vi "EVO_main_raw_dev_MQTTT_RT_raw.vi"() -> ()   [LabVIEW 2017]
uses:
  controls/FPGA State.ctl
  mqtt Folder/src/class/mqtt/mqttTypedef/mqttConnectionStatus.ctl
  mqtt Folder/src/class/mqtt/mqttTypedef/mqttConnectionMeta.ctl
  mqtt Folder/src/class/mqtt/mqttTypedef/mqttQOSlevel.ctl
  controls/UI Data2.ctl
  mqtt Folder/src/class/mqtt/mqttTXqueue/mqttTXdataQueueFunction.ctl
  mqtt Folder/src/class/mqtt/mqttConfigFunction.ctl
  mqtt Folder/src/class/mqtt/mqttTypedef/mqttConnectionFlags.ctl
  mqtt Folder/src/class/mqtt/mqttTypedef/mqttWillInformation.ctl
  mqtt Folder/src/class/mqtt/mqttTypedef/mqttBroker.ctl
  controls/Chatter data.ctl
  <vilib>/addons/database/Connection.llb/DB Tools Open Connec (Path).vi
  Globals/Global - All UI Loop Stop.vi
  Globals/Global - UI Stream and Variable Connections.vi
  Globals/Global - Configuration Options.vi
  UI Error Handlers/support/User Event - Stop/User Event - Stop.lvlib
  UI Error Handlers/support/Message Queue/Message Queue.lvlib
  mqtt Folder/src/class/mqtt/mqtt.lvclass
  <vilib>/addons/database/NI_Database_API.lvlib
panel:
  out "size(s) 2":i32
  out "size(s)":i32
  out "publishSuccess":bool=TRUE
  out "publishMessageID":u16 format="%02x"
  in  "connMeta":T1
  in  "topic":string="a/b"
  out "connStatus 2":T3
  out "success":bool
  out "sessionPresent 2":bool
  in  "error in (no error)":errorcluster
  out "tag spike":string
  out "string":string
  out "x .or. y?":bool
  out "resulting string":string
  in  "Settings Tab":T4(tab)=enum."Sensor data "
  in  "Database_machine":string="Raw.DMG_MORI_DMU_40_EVO_RAW"
  in  "OK Button":bool
  in  "Tool Data File":path=path "K:/Core Research/Project Folders/AI Projects/AI3190 Digital Shop Floor Rollout/5 Software Files/Catapult/tool_path.txt"
  in  "Run Control":bool
  in  "Stop Control":bool
  in  "Max Acceleration Threshold (g)":sgl=0.03
  in  "In-cut Power Threshold":dbl=1.0
  in  "Controller Address":string="127.22.11.2"
  in  "Connect to Controller":bool
  out "Connected?":bool
  out "System Status":string
  in  "Save?":bool
  in  "Switch to Safe State":bool
  out "Current FPGA State":T5
  out "Tool Data":string="\n"
  in  "ODBC data source name":string="amrc_monitoring"
  in  "MT Connect Agent":string="http://amrcmtconnect.shef.ac.uk:5000/"
  in  "milliseconds to wait":u32=100
  in  "Machine":string="DMU40EVO"
  out "Loop execution":u32
  out "output cluster":cluster{"G1 ":bool}
  out "Chatter?":bool
  out "Automated FRF  (grms) 2":T6(graph)
  out "ACC  (grms)":T7(graph)
  out "Strain (grms)":T8(graph)
  out "Raw ACC":waveform(dbl)[](graph)
  out "Raw Waveform 2":waveform(dbl)[](graph)
  out "tag acc":string
  out "Feed rate":dbl[](graph)
  out "Spindle Speed":dbl[](graph)
  out "Spindle Load":dbl[](graph)
  out "H5 machine":bool
  out "Tool id":string
  out "RPM":dbl
  out "Program Name":string
  out "Block of code being executed":string
  out "Feed":dbl
  out "CPU Usage (%)":dbl[][](graph)
  out "Free Physical Memory or Largest Contiguous Memory (bytes)":dbl(graph)
  out "DMA FIFO Overflow?":bool
  in  "Exit":bool
  # "Acceleration Waveform for 0.5s"
  # "Connection Settings"
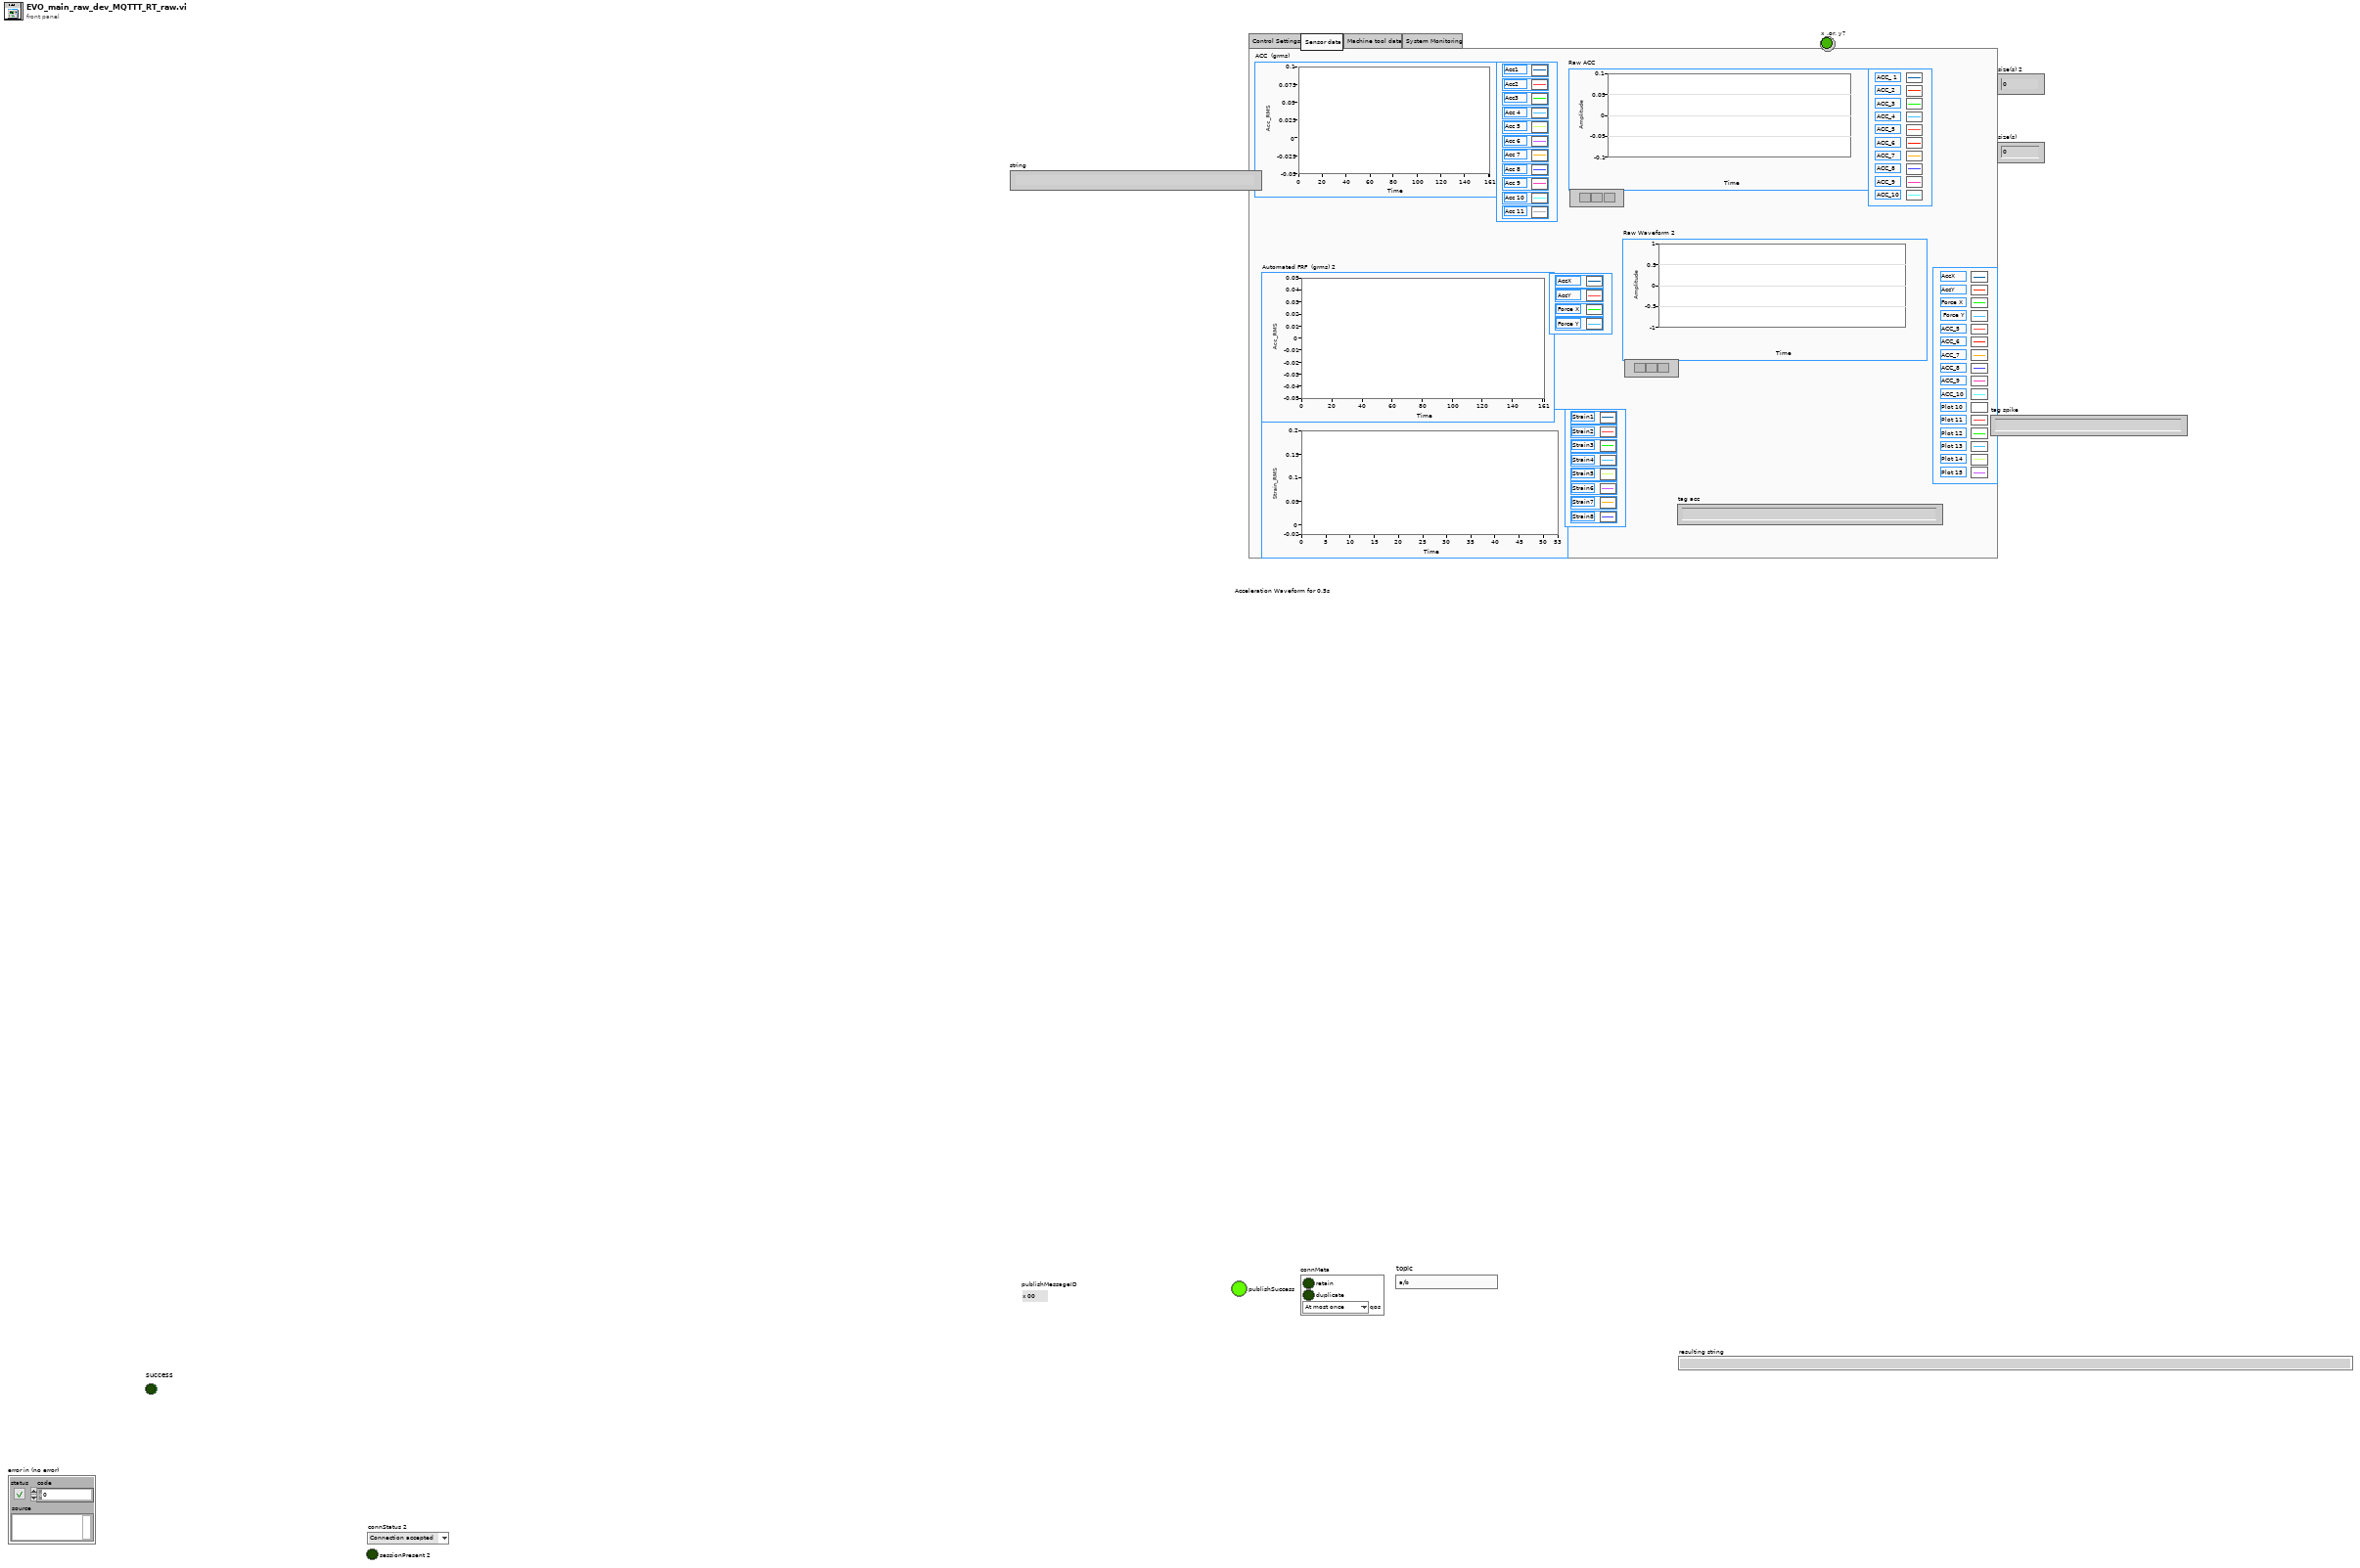
[diagram p1: front panel]
types:
  T1 = typedef "mqttConnectionMeta.ctl" = cluster{"retain":bool, "duplicate":bool, "qos":T2}
  T2 = typedef "mqttQOSlevel.ctl" = enum8{"At most once", "At least once", "Exactly once", "Reserved"}
  T3 = typedef "mqttConnectionStatus.ctl" = enum16{"Connection accepted", "Connection refused: unacceptable protocol version", "Connection refused: identifier rejected", "Connection refused: Server unavailable", "Connection refused: bad user name or password", "Connection refused: not authorized"}
  T4 = enum32{"Control Settings", "Sensor data ", "Machine tool data", "System Monitoring"}
  T5 = typedef "FPGA State.ctl" = enum16{"Safe State", "Control (PID)"}
  T6 = cluster{"[0]":dbl, "[1]":dbl, "[2]":dbl, "[3]":dbl}
  T7 = cluster{"[0]":dbl, "[1]":dbl, "[2]":dbl, "[3]":dbl, "[4]":dbl, "[5]":dbl, "[6]":dbl, "[7]":dbl, "[8]":dbl, "[9]":dbl, "[10]":dbl}
  T8 = cluster{"[0]":dbl, "[1]":dbl, "[2]":dbl, "[3]":dbl, "[4]":dbl, "[5]":dbl}
  T9 = typedef "mqttBroker.ctl" = cluster{"address":string, "port":u16, "connTimeout":i32, "writeTimeout":i32, "readTimeout":i32, "subTimeout":i32}
  T10 = typedef "mqttWillInformation.ctl" = cluster{"User Name":string, "Password":string}
  T11 = typedef "mqttConnectionFlags.ctl" = cluster{"reserved":bool, "clean session":bool, "will flag":bool, "willQOS":enum8{"At most once", "At least once", "Exactly once", "Reserved"}, "will retain":bool, "password":bool, "user name":bool}
  T12 = typedef "mqtt.lvclass/mqttConfigFunction.ctl" = enum16{"init", "deinit", "set", "get"}
  T13 = enum8{"Enabled", "Disabled", "Disabled and Grayed Out"}
  T14 = typedef "mqttTXdataQueueFunction.ctl" = enum16{"init", "deinit", "getQueue", "enqueue"}
  T15 = typedef "UI Data2.ctl" = cluster{"Switch to Safe State Ref":refnum<vi>, "Run Control Ref":refnum<vi>, "Stop Control Ref":refnum<vi>, "Update Control Configurations Ref":refnum<vi>, "Chatter Data Ref":refnum<vi>, "Max Acceleration Threshold Ref":refnum<vi>}
  T16 = typedef "NI_Database_API.lvlib/Conn ObjectReference.ctl" = refnum<k1>
  T17 = typedef "Message Queue.lvlib/All Message Queues.ctl" = cluster{"UI":refnum<queue>}
  T18 = cluster{"Message":string, "Message Data":variant}
  T19 = typedef "Chatter data.ctl" = cluster{"Tool data":cluster{"Number of teeth":sgl}, "Cutting data":cluster{"rpm":sgl}, "Limits":cluster{"Magnitude threshold":sgl, "Tolerance":sgl}, "G1 status":cluster{"G1 ":bool}}
  T20 = cluster{"FPGA State":T5, "Max Acceleration Threshold":sgl, "Chatter Data":T19}
  T21 = cluster{"seconds since 1Jan1904":timestamp, "number":dbl[][], "Machine Data":cluster{"Zload":string, "Yload":string, "Xload":string, "path_position":string, "Fovr":string, "SspeedOvr":string, "Program Name":string, "Program status":string, "Block of code being executed":string, "Line of code":string, "Machine availability":string, "Emergency status":string, "Controller mode":string, "Tool_id":string}}
  T22 = cluster{"seconds since 1Jan1904":timestamp, "number":dbl[][], "Machine Data":cluster{"Zload":string, "Yload":string, "Xload":string, "path_position":string, "Fovr":string, "SspeedOvr":string, "Program Name":string, "Program status":string, "Block of code being executed":string, "Line of code":string, "Machine availability":string, "Emergency status":string, "Controller mode":string, "Tool id":string}}
  T23 = cluster{"Actual PID Loop Period":refnum<k21>, "DMA FIFO Overflow?":refnum<k21>, "CPU Usage":refnum<k21>, "Free or Contiguous Memory":refnum<k21>, "Current FPGA State":refnum<k21>, "Acceleration (grms)":refnum<k21>, "Acceleration Waveform":refnum<k21>, "Chatter":refnum<k21>, "tag acc":refnum<k21>, "tag video":refnum<k21>, "Image Waveform":refnum<k21>}
  T24 = cluster{"Zload":string, "Yload":string, "Xload":string, "path_position":string, "Fovr":string, "SspeedOvr":string, "Program Name":string, "Program status":string, "Block of code being executed":string, "Line of code":string, "Machine availability":string, "Emergency status":string, "Controller mode":string, "Tool_id":string}
  T25 = cluster{"Zload":string, "Yload":string, "Xload":string, "path_position":string, "Fovr":string, "SspeedOvr":string, "Program Name":string, "Program status":string, "Block of code being executed":string, "Line of code":string, "Machine availability":string, "Emergency status":string, "Controller mode":string, "Tool id":string}
  T26 = cluster{"Magnitude threshold":sgl, "Tolerance":sgl}
  T27 = typedef "FPGA state.ctl" = enum16{"Safe State", "Control (PID)"}
  T28 = typedef "IMAQ Image.ctl" = refnum<image>
  T29 = typedef "CPU Loads.ctl" = cluster{"Total (%)":dbl, "Time Critical (%)":dbl, "Timed Structures (%)":dbl, "High (%)":dbl, "Above Normal (%)":dbl, "Normal (%)":dbl, "Background (%)":dbl, "Idle (%)":dbl, "ISR (%)":dbl}[]
  T30 = cluster{"seconds since 1Jan1904":timestamp, "appended array":dbl[][], "Machine Data":cluster{"Zload":string, "Yload":string, "Xload":string, "path_position":string, "Fovr":string, "SspeedOvr":string, "Program Name":string, "Program status":string, "Block of code being executed":string, "Line of code":string, "Machine availability":string, "Emergency status":string, "Controller mode":string, "Tool_id":string}}
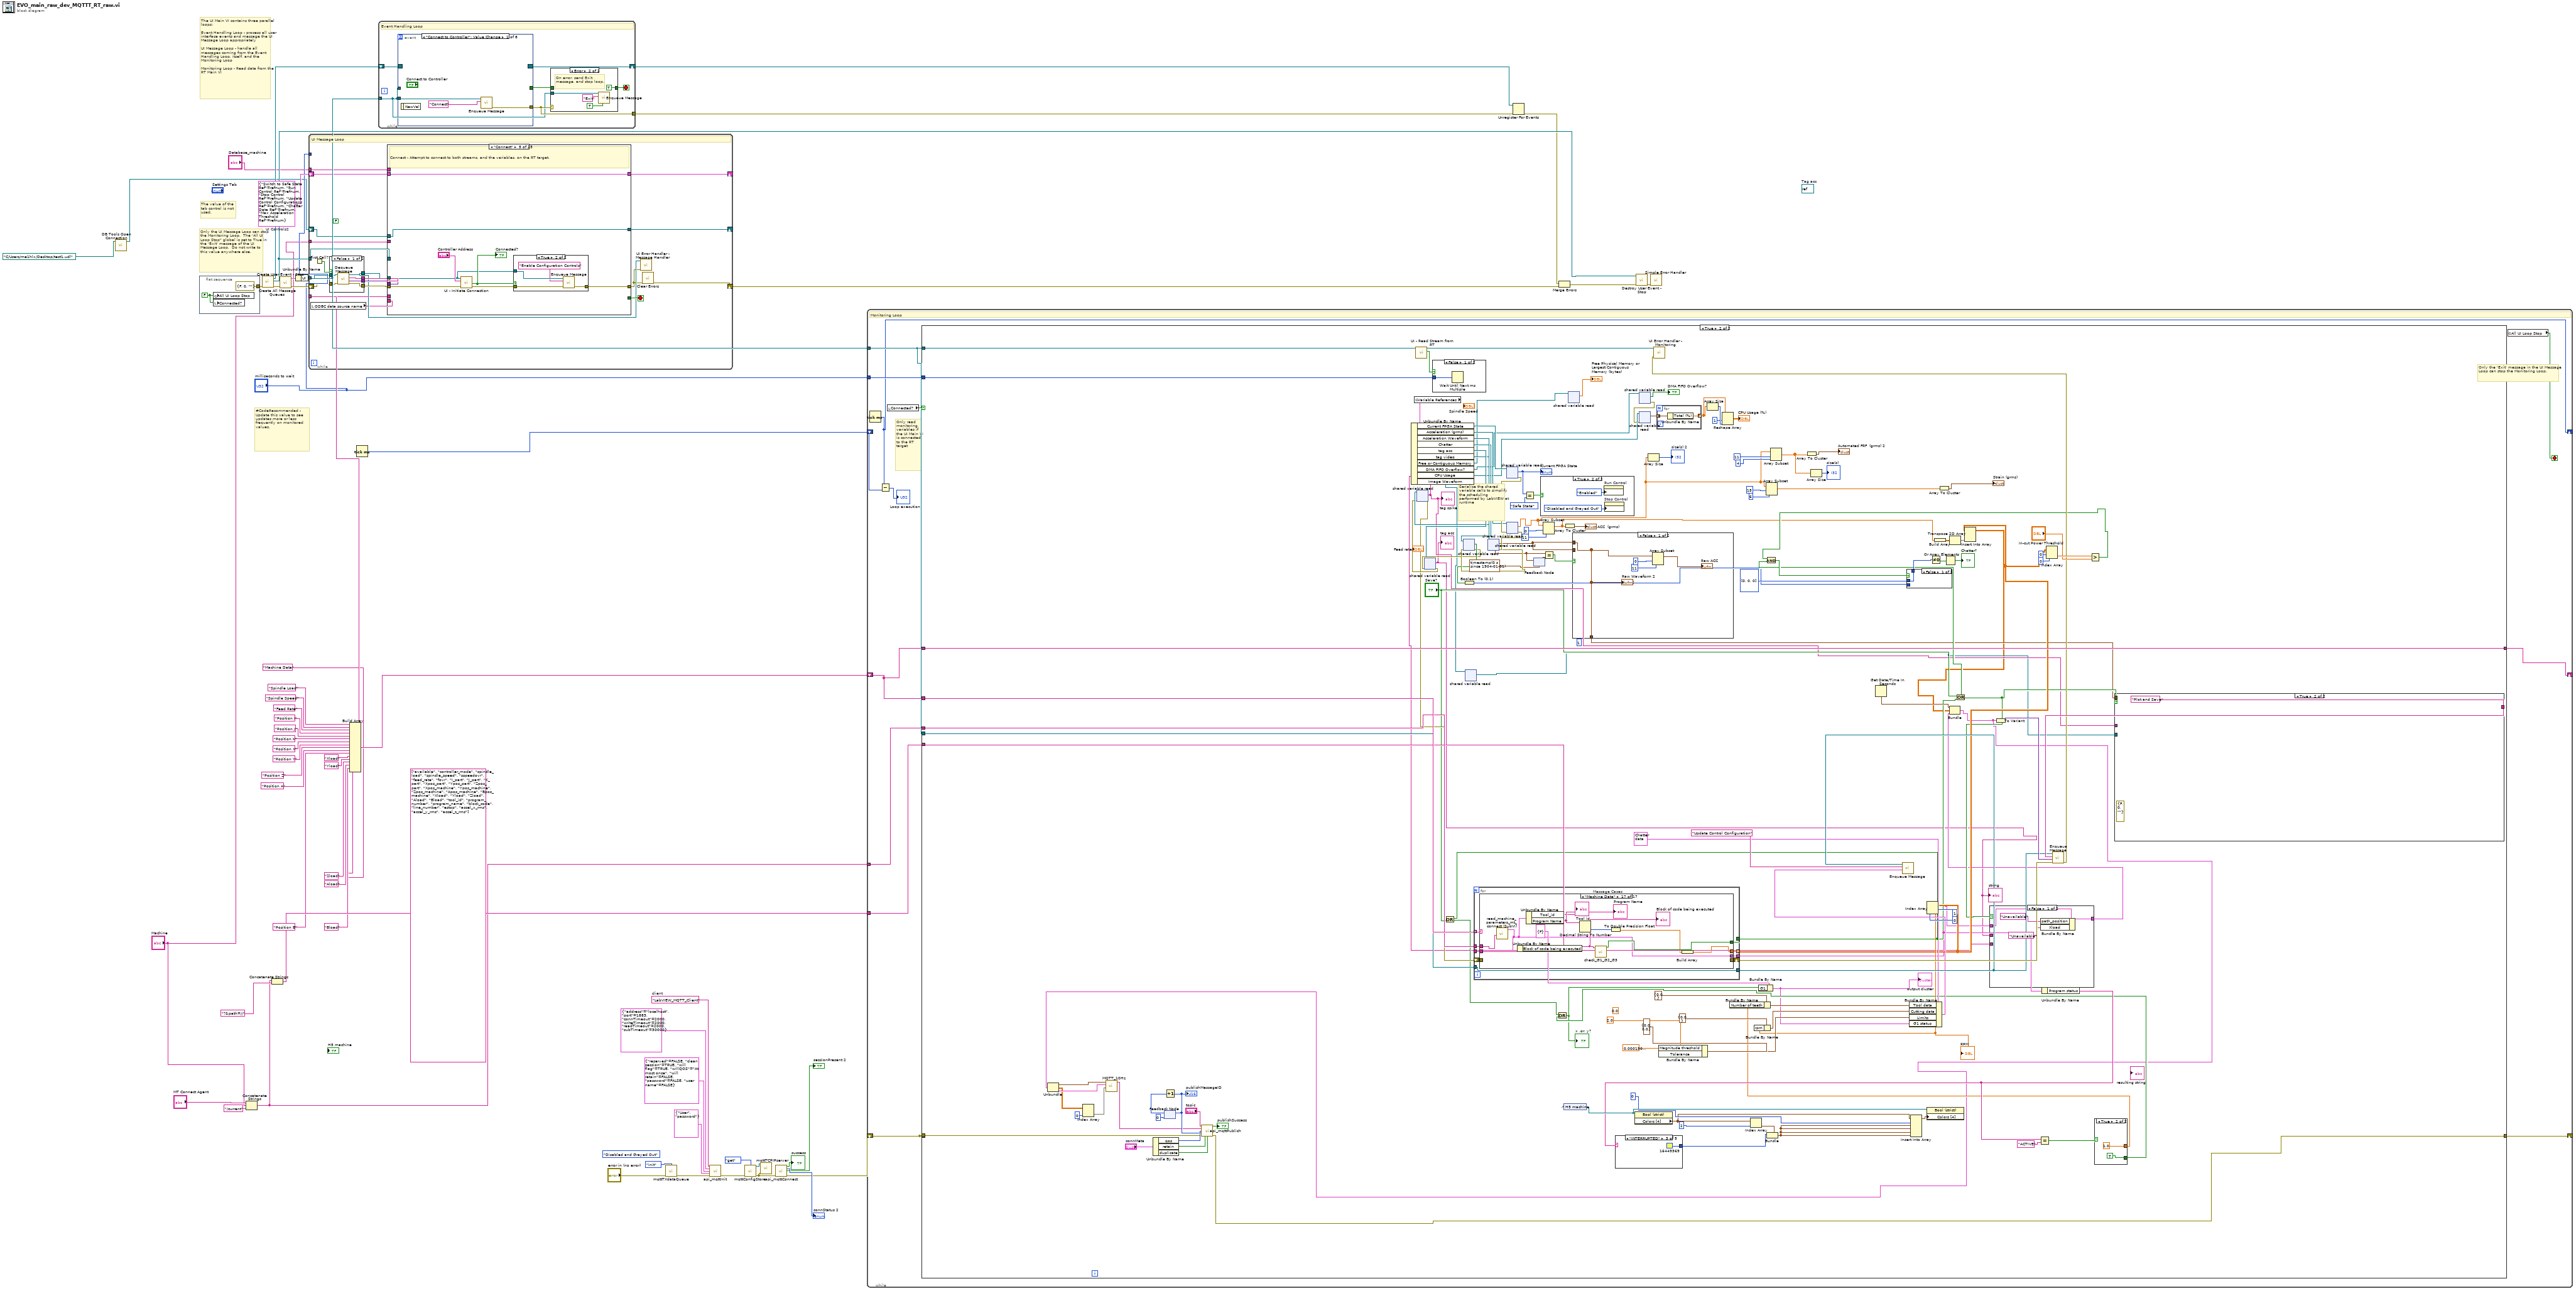
[diagram p0: block diagram]
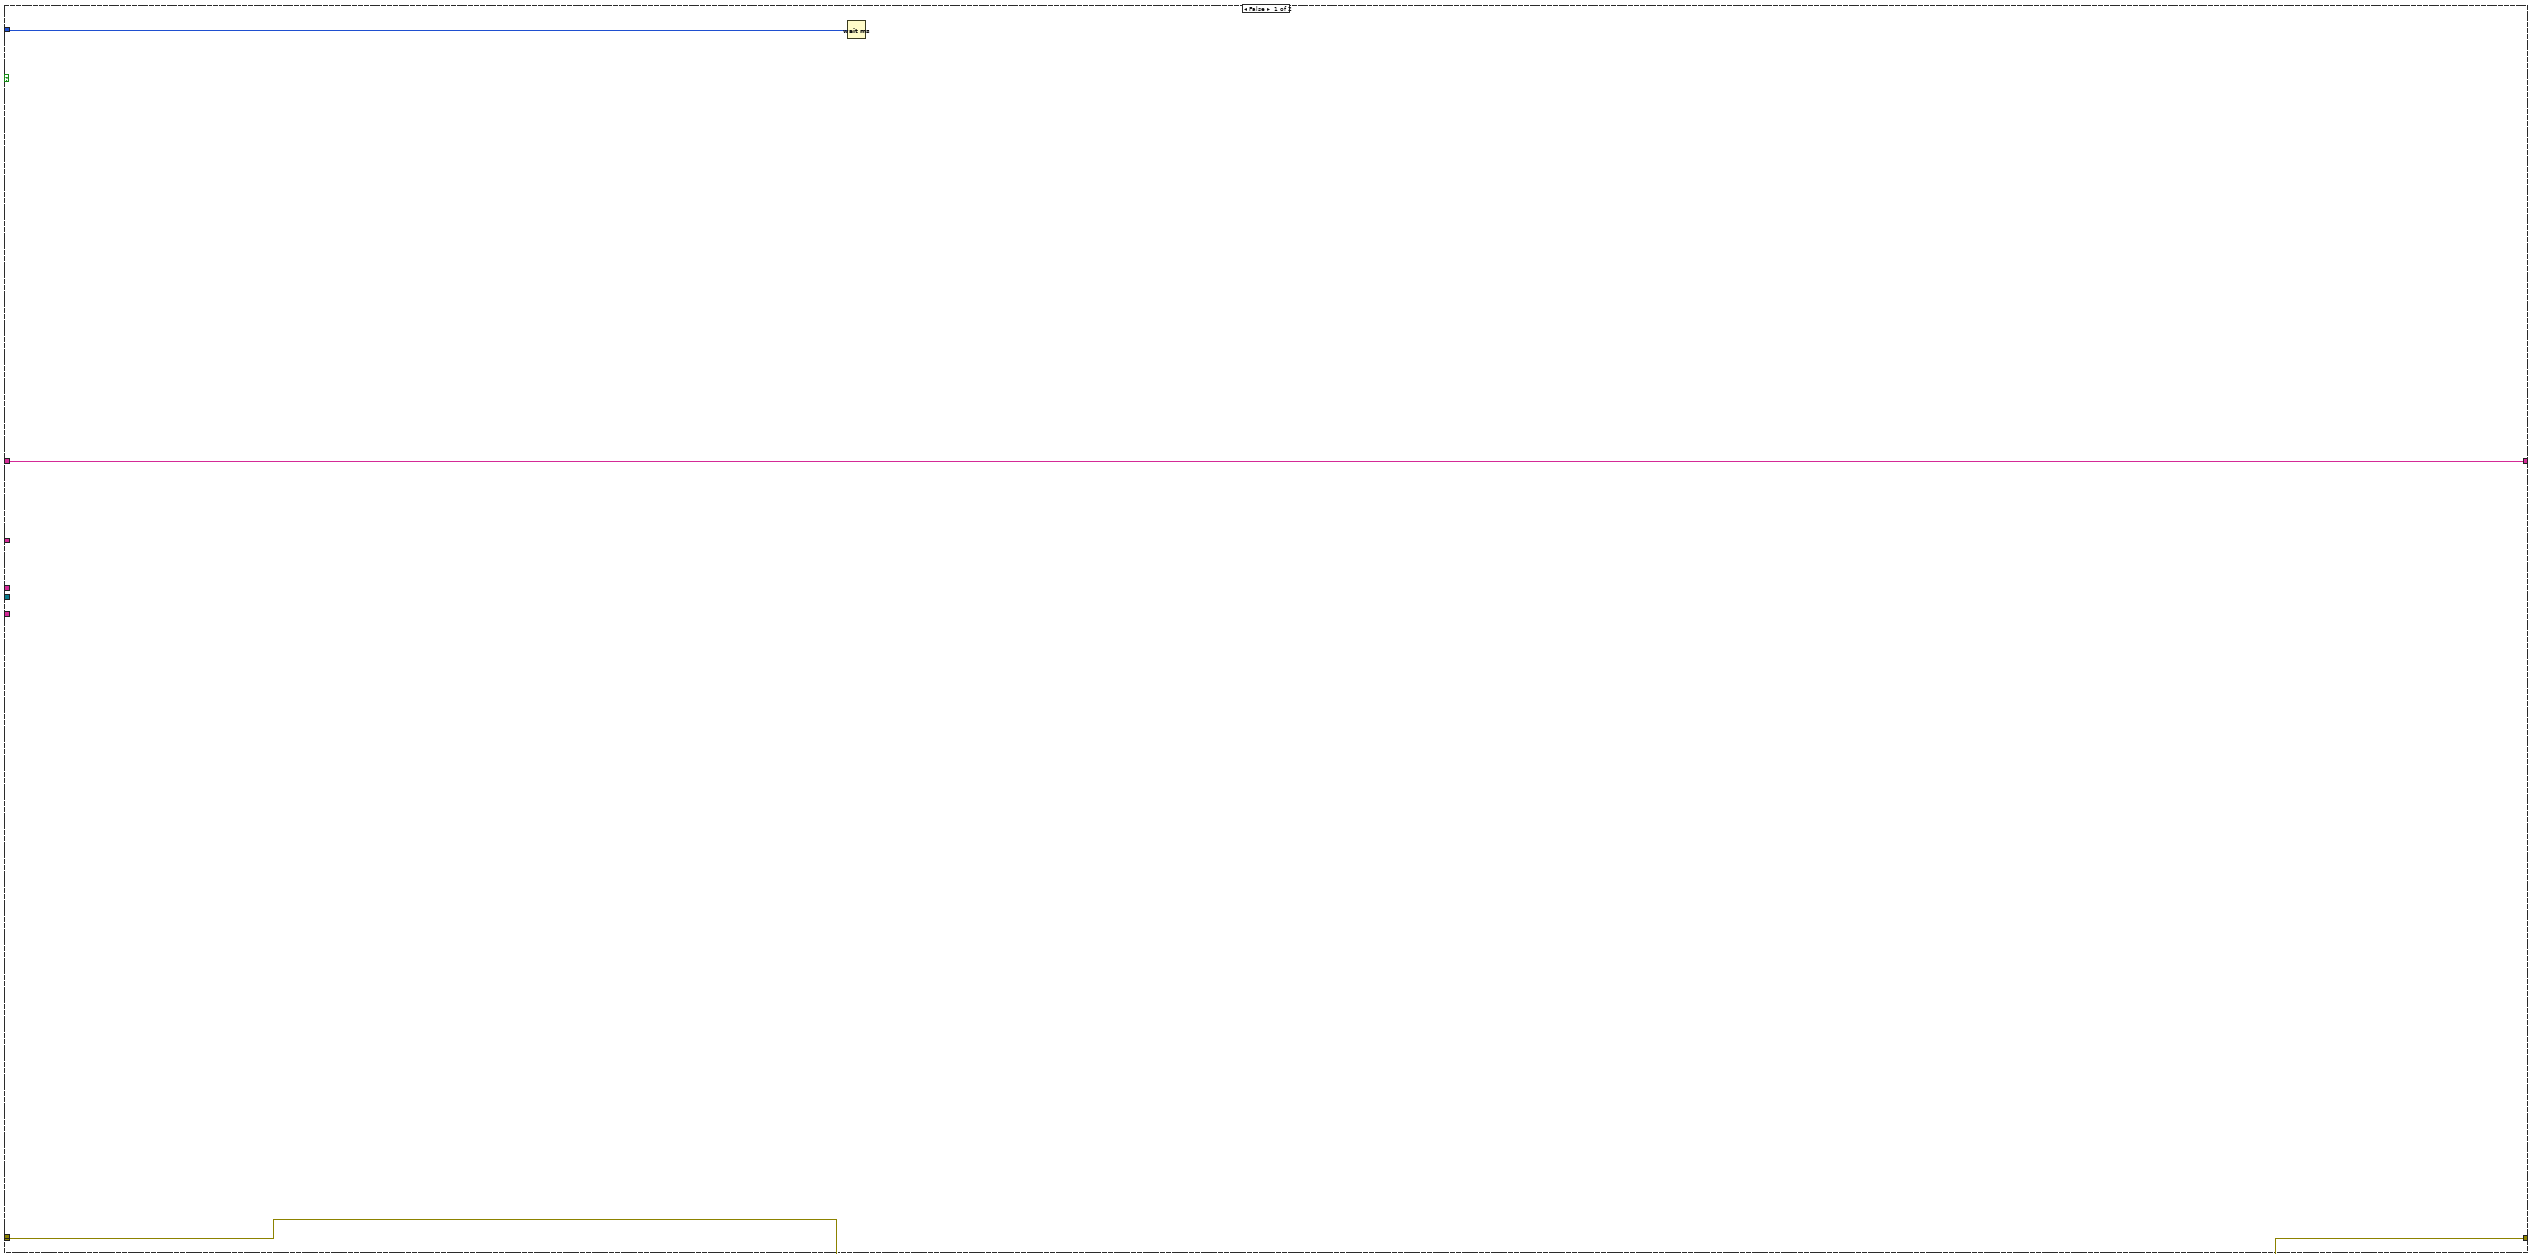
[diagram p2: hidden frame]
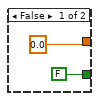
[diagram p3: hidden frame]
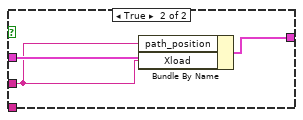
[diagram p4: hidden frame]
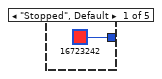
[diagram p5: hidden frame]
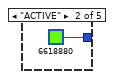
[diagram p6: hidden frame]
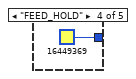
[diagram p7: hidden frame]
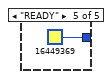
[diagram p8: hidden frame]
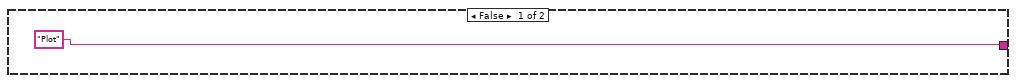
[diagram p10: hidden frame]
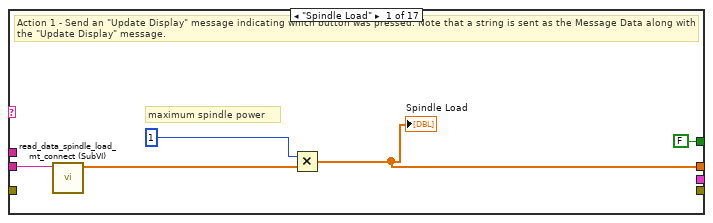
[diagram p11: hidden frame]
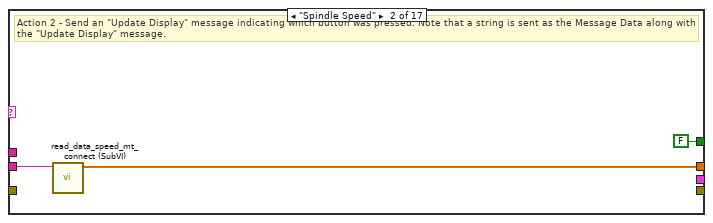
[diagram p12: hidden frame]
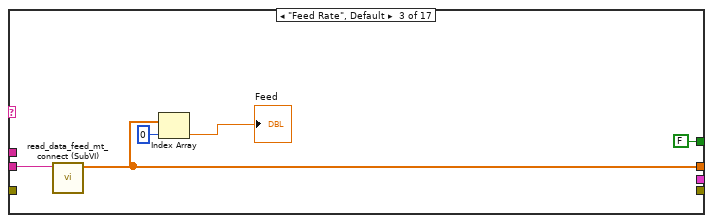
[diagram p13: hidden frame]
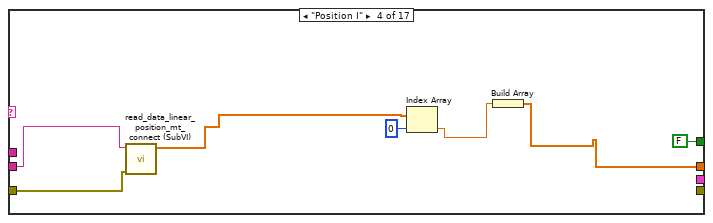
[diagram p14: hidden frame]
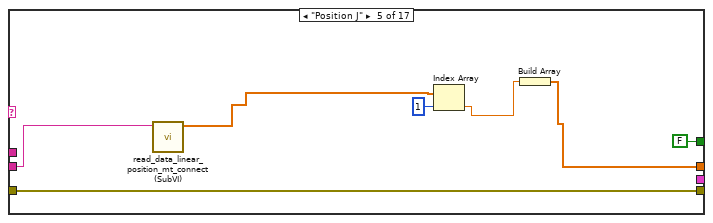
[diagram p15: hidden frame]
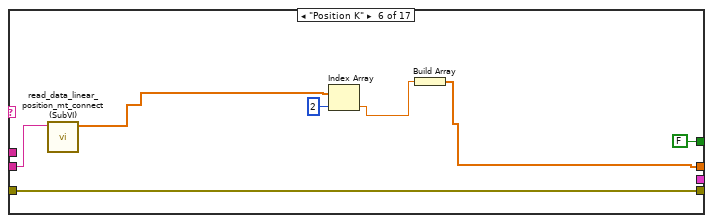
[diagram p16: hidden frame]
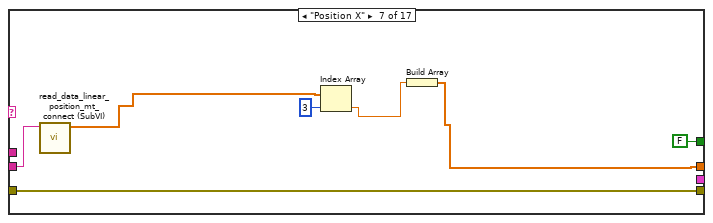
[diagram p17: hidden frame]
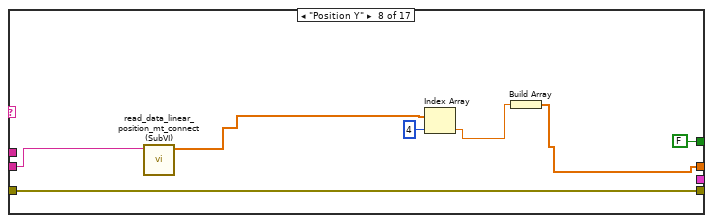
[diagram p18: hidden frame]
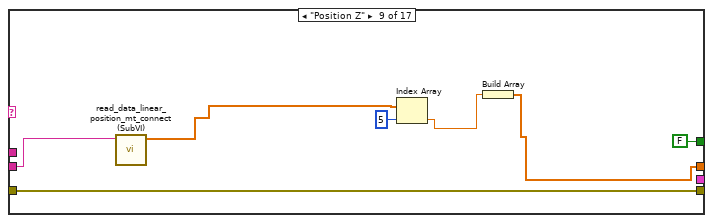
[diagram p19: hidden frame]
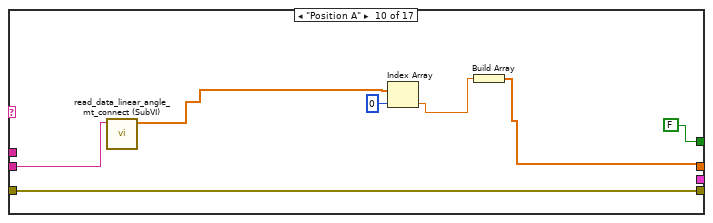
[diagram p20: hidden frame]
diagram:
  w8 = "LabVIEW_MQTT_Client"  # client
  (unwired) T13."Disabled and Grayed Out" ("Disabled")
  (unwired) string[] ["available", "controller_mode", "spindle_load", "spindle_speed", "sspeedovr", "feed_rate", "fovr", "I_part", "J_part", "K_part", "Xpos_part", "Ypos_part", "Zpos_part", "Xpos_machine", "Ypos_machine", "Zpos_machine", "Apos_machine", "Bpos_machine", "Xload", "Yload", "Zload", "Aload", "Bload", "tool_id", "program_number", "program_name", "block_code", "line_number", "estop", "accel_x_rms", "accel_y_rms", "accel_z_rms"]
  (unwired) refnum<k21> refnum  # Tag acc
  (unwired) FALSE ("Record  SS 661")
  w45 = T15 {"Switch to Safe State Ref"=refnum, "Run Control Ref"=refnum, "Stop Control Ref"=refnum, "Update Control Configurations Ref"=refnum, "Chatter Data Ref"=refnum, "Max Acceleration Threshold Ref"=refnum}  # UI Controls2
  # "#CodeRecommended - Update this value to see updates more or less frequently on monitored values."
  # "The UI Main VI contains three parallel loops:\n\nEvent Handling Loop - process all user interface events and message the UI Message Loop appropriately\n\nUI Message Loop - handle all messages coming from the Event Handling Loop, itself, and the Monitoring Loop\n\nMonitoring Loop - Read data from the RT Main VI"
  # "The value of the tab control is not used."
  # "Only the UI Message Loop can stop the Monitoring Loop.  The 'All UI Loop Stop\" global is set to True in the 'Exit' message of the UI Message Loop.  Do not write to this value anywhere else."
  n1 = call-poly <vilib>:"DB Tools Open Connection.vi"("connection information"=path "C:/Users/me1hlx/Desktop/test1.udl") -> ("connection reference"=w1:T16)  [unwired: 7 in, 1 out]
  n2 = flat-sequence {
    tunnel: [errorcluster {"status"=FALSE, "code"=0, "source"=""} ("error in (no error)")] -> w46
    frame #0 {
      w59 = FALSE
      n3 = global write "Global - All UI Loop Stop.vi" "All UI Loop Stop"(w59) -> ()
      n4 = local write "Connected?"(w59) -> ()
    }
  }
  n5 = Concatenate Strings("MT Connect Agent", "Machine", "/current" ("string")) -> (w36:string)
  n6 = call "Create User Event - Stop.vi"("error in (no error)"=w46) -> ("error out"=w53:errorcluster, "User Event - Stop"=w54:refnum<user-event>, "Stop Event Registration Refnum"=w55:refnum<event-registration>)  [unwired: 8 in]
  n7 = Concatenate Strings(w36, "?&path=//" ("string")) -> (w40:string)
  n8 = call "Create All Message Queues.vi"("error in (no error)"=w53) -> ("error out"=w51:errorcluster, "Message Queues out"=w52:T17)  [unwired: 9 in]
  n9 = Unbundle By Name(w52) -> ("UI"=w47:refnum<queue>)
  n10 = Build Array("Spindle Load" ("Message"), "Spindle Speed" ("Message"), "Feed Rate" ("element"), "Position I" ("element"), "Position J" ("element"), "Position K" ("element"), "Position X" ("element"), "Position Y" ("element"), "Position Z" ("element"), "Position A" ("element"), "Position B" ("element"), "Xload" ("element"), "Yload" ("element"), "Zload" ("element"), "Aload" ("element"), "Bload" ("element"), "Machine Data" ("element")) -> (w39:string[])
  n11 = while {
    tunnel: w47 -> [w73]
    tunnel: w54 -> [w78]
    shift-right: [w68] -> w58
    shift-left: w51 -> [w77]
    shift-right: [w71] -> _
    shift-left: w45 -> [w72]
    tunnel: w39 -> [w67]
    tunnel: "Machine" -> [w66]
    tunnel: "milliseconds to wait" -> [_]
    tunnel: "Database_machine" -> [w64]
    shift-right: [w62] -> _
    shift-left: w1 -> [w63]
    stop <- w79 stop-if-true
    # "UI Message Loop"
    n12 = local read "ODBC data source name"() -> (w65:string)
    n13 = First Call?() -> (First Call?: T/F=w61:bool)
    n14 = case shown="False" w61 {
      tunnel: w77 -> [w85 w86]
      tunnel: [w84 w86] -> w76
      tunnel: [w83 "Connect" ("Message")] -> w75
      tunnel: [w82 _] -> w74
      tunnel: w73 -> [w81 w87]
      tunnel: [w80 w87] -> w70
      frame False {
        n15 = call "Dequeue Message.vi"("error in (no error)"=w85, "Message Queue"=w81) -> ("error out"=w84:errorcluster, "Message Data"=w82:variant, "Message"=w83:string, "dup Message Queue"=w80:refnum<queue>)  [unwired: 6 in]
      }
      frame True {
      }
    }
    n16 = case "Message Cases" shown="\"Connect\"" w75 {
      selector: w75 -> [_ _ _ _ _ _ _ _ _ _ _ _ w234 _ w270 _ w307 _ _ _ _ _ w412]
      tunnel: w70 -> [w91 w98 _ _ w134 _ w154 w163 _ w190 _ _ w235 _ _ _ w311 _ w356 _ _ w385 _]
      tunnel: w76 -> [w93 w105 w119 w126 w139 w151 w156 w161 w178 w199 w215 w230 w237 w256 w271 w290 w321 w343 w361 w367 w380 w386 _]
      tunnel: [w92 w99 w119 w126 w133 w151 w155 w166 w177 w192 w208 w222 w236 w258 w272 w289 w322 w341 w362 w366 w379 w389 w410] -> w69
      tunnel: [_ _ _ _ _ _ _ _ _ _ _ _ _ _ _ _ _ _ TRUE _ _ _ _] -> w79
      tunnel: w74 -> [_ _ _ _ _ _ _ _ _ w197 w214 w229 _ w255 w269 w288 w319 w340 _ _ w377 _ _]
      tunnel: w78 -> [_ _ _ _ _ _ _ _ _ _ _ _ _ _ _ _ _ _ w360 _ _ _ _]
      tunnel: w72 -> [w94 w104 w118 w128 w138 w150 w158 w167 w179 w195 w216 w231 w238 w259 w273 w287 w323 w342 w358 w365 w378 w388 w408]
      tunnel: [w94 w103 w118 w128 w138 w150 w158 w167 w179 w195 w216 w231 w238 w259 w273 w287 w323 w342 w358 w365 w378 w388 w408] -> w71
      tunnel: w67 -> [_ _ _ _ _ _ _ _ _ _ _ _ _ _ _ _ _ _ _ _ _ _ _]
      tunnel: w65 -> [_ _ _ _ _ _ _ _ _ _ _ _ _ _ _ _ _ _ _ _ _ _ _]
      tunnel: w66 -> [_ _ _ _ _ _ _ _ _ _ _ _ _ _ _ _ _ _ _ _ _ _ _]
      tunnel: w64 -> [_ _ _ _ _ _ _ _ _ _ w205 w219 _ _ _ _ _ _ _ _ _ _ _]
      tunnel: w63 -> [w89 w95 w106 w120 w132 w145 w152 w159 w175 w185 w203 w218 w232 w252 w267 w281 w305 w331 w350 w364 w368 w383 w407]
      tunnel: [w89 w95 w106 w120 w132 w145 w152 w159 w175 w185 w204 w217 w232 w252 w267 w281 w305 w331 w350 w364 w368 w383 w407] -> w62
      frame "Initialize" {
        # "Initialize - Send 'Initialize UI Refs' message to get the UI references bundled and initialized appropriately."
        n17 = call "Enqueue Message.vi"("error in (no error)"=w93, "Message"="Initialize UI Refs", "Message Queue"=w91) -> ("error out"=w92:errorcluster)  [unwired: 7 in, 1 out]
      }
      frame "Initialize UI Refs" {
        # "Send a message to disable them all, since there is no connection at the start."
        # "Initialize UI Refs - Bundle up a cluster of references of all UI elements that are programmatically manipulated."
        n18 = control-ref of="Max Acceleration Threshold (g)"() -> (w96:refnum<vi>)
        n19 = control-ref of="Switch to Safe State"() -> (w102:refnum<vi>)
        n20 = control-ref of="Run Control"() -> (w101:refnum<vi>)
        n21 = control-ref of="Stop Control"() -> (w100:refnum<vi>)
        n22 = call "Enqueue Message.vi"("error in (no error)"=w105, "Message"="Disable Controls", "Message Queue"=w98) -> ("error out"=w99:errorcluster)  [unwired: 7 in, 1 out]
        n23 = Bundle By Name(cluster=w104, "Switch to Safe State Ref"=w102, "Run Control Ref"=w101, "Stop Control Ref"=w100, "Max Acceleration Threshold Ref"=w96) -> (w103:T15)
      }
      frame "Disable Controls" {
        w109 = 0
        # "With the control options disabled, the only thing the user can do is Connect. Make sure the IP address string and connect button are enabled."
        # "Disable All Controls - Set all controls in the UI Refs cluster to \"Disabled and Grayed Out\"."
        n24 = Unbundle(w118) -> ("Switch to Safe State Ref"=w117:refnum<vi>, "Run Control Ref"=w116:refnum<vi>, "Stop Control Ref"=w115:refnum<vi>, "Update Control Configurations Ref"=w114:refnum<vi>, "Chatter Data Ref"=w113:refnum<vi>, "Max Acceleration Threshold Ref"=w112:refnum<vi>)
        n25 = Build Array(w117, w116, w115, w114, w113, w112) -> (w111:refnum<vi>[])
        n26 = property on="ODBC data source name" class="Str"("DisabledEnum"=T13."Enabled" ("Disabled")) -> ()  [unwired: 2 in, 2 out]
        n27 = property on="In-cut Power Threshold" class="DigNum (strict)"("DisabledEnum"=T13."Disabled and Grayed Out" ("Disabled")) -> ()  [unwired: 2 in, 2 out]
        n28 = call "Set Enable State on Multiple Controls.vi"("Enable?"=FALSE, "Controls"=w111) -> ()  [unwired: 10 in]
        n29 = property on="Controller Address" class="Str"("DisabledEnum"=w109) -> ()  [unwired: 2 in, 2 out]
        n30 = property on="Connect to Controller" class="Bool"("DisabledEnum"=w109) -> ()  [unwired: 2 in, 2 out]
      }
      frame "Enable Configuration Controls" {
        w129 = 2
        # "Once connected, the user shouldn't be able to change the connection settings unless he gets disconnected."
        # "Enable Configuration Controls - After successful connection, ensure appropriate controls are enabled."
        n31 = Unbundle By Name(w128) -> ("Update Control Configurations Ref"=w127:refnum<vi>, "Max Acceleration Threshold Ref"=w125:refnum<vi>, "Chatter Data Ref"=w124:refnum<vi>, "Switch to Safe State Ref"=w123:refnum<vi>)
        n32 = property on="In-cut Power Threshold" class="DigNum (strict)"("DisabledEnum"=T13."Enabled" ("Disabled")) -> ()  [unwired: 2 in, 2 out]
        n33 = property on="ODBC data source name" class="Str"("DisabledEnum"=T13."Disabled and Grayed Out" ("Disabled")) -> ()  [unwired: 2 in, 2 out]
        n34 = Build Array(w127, w125, w124, w123) -> (w131:refnum<vi>[])
        n35 = call "Set Enable State on Multiple Controls.vi"("Enable?"=TRUE, "Controls"=w131) -> ()  [unwired: 10 in]
        n36 = property on="Controller Address" class="Str"("DisabledEnum"=w129) -> ()  [unwired: 2 in, 2 out]
        n37 = property on="Connect to Controller" class="Bool"("DisabledEnum"=w129) -> ()  [unwired: 2 in, 2 out]
      }
      frame "Connect" {
        # "Connect - Attempt to connect to both streams, and the variables, on the RT target."
        n38 = call "UI - Initiate Connection.vi"("error in (no error)"=w139, "Controller Address"="Controller Address", "Message Queue"=w134) -> ("error out"=w136:errorcluster, "Connected?"=w135:bool)  [unwired: 7 in]
        "Connected?" <- w135
        n39 = case shown="True" w135 {
          tunnel: w136 -> [w140 w144]
          tunnel: w134 -> [_ w143]
          tunnel: [w140 w142] -> w133
          frame False {
          }
          frame True {
            n40 = call "Enqueue Message.vi"("error in (no error)"=w144, "Message"="Enable Configuration Controls", "Message Queue"=w143) -> ("error out"=w142:errorcluster)  [unwired: 7 in, 1 out]
          }
        }
      }
      frame "Close Connections" {
        # "Close Connections - Close the connections shared with the Monitoring Loop."
        n41 = global read "Global - UI Stream and Variable Connections.vi" "UI Command Stream"() -> (w149:refnum<k21>)
        n42 = global read "Global - UI Stream and Variable Connections.vi" "RT Message Stream"() -> (w148:refnum<k21>)
        n43 = global read "Global - UI Stream and Variable Connections.vi" "Variable References"() -> (w146:T23)
        n44 = local write "Connected?"(FALSE ("Connected?")) -> ()
        n45 = Destroy Stream Endpoint(11:w149) -> ()  [unwired: 1 in, 1 out]
        n46 = Destroy Stream Endpoint(11:w148) -> ()  [unwired: 1 in, 1 out]
        n47 = call "Close Variable Connections.vi"("Variable References 2"=w146) -> ()  [unwired: 11 in]
      }
      frame "Disconnect UI" {
        # "Disable Controls"
        # "Disconnect UI - Something has gone wrong with the connection. Reinitialize the UI to its disconnected state."
        n48 = local write "Connected?"(FALSE ("Connected?")) -> ()
        n49 = call "Enqueue Message.vi"("error in (no error)"=w156, "Message"="Reconnect", "Message Queue"=w154) -> ("error out"=w155:errorcluster)  [unwired: 7 in, 1 out]
      }
      frame "Reconnect" {
        # "Disconnect UI - Something has gone wrong with the connection. Reinitialize the UI to its disconnected state."
        n50 = Flush Queue(queue=w163, error in (no error)=w161) -> (queue out=w162:refnum<queue>, error out=w160:errorcluster)  [unwired: 1 out]
        n51 = flat-sequence {
          tunnel: w162 -> [w169]
          tunnel: w160 -> [w170]
          tunnel: [w170] -> w165
          tunnel: [w169] -> w164
          tunnel: w165 -> [w173]
          tunnel: w164 -> [w171]
          tunnel: [w172] -> w166
          frame #0 {
            n52 = Wait Until Next ms Multiple(millisecond multiple=u32 10000) -> ()  [unwired: 1 out]
          }
          frame #1 {
            n53 = call "Enqueue Message.vi"("error in (no error)"=w173, "Message"="Connect", "Message Queue"=w171) -> ("error out"=w172:errorcluster)  [unwired: 7 in, 1 out]
          }
        }
      }
      frame "Get Settings from FPGA" {
        # "Get Settings from FPGA - Send a command to the RT to retrieve all current FPGA Main VI parameter values and send them back to the UI."
        n54 = local read "Connected?"() -> (w176:bool)
        n55 = case shown="True" w176 {
          tunnel: w178 -> [w180 w184]
          tunnel: [w180 w183] -> w177
          frame False {
            # "Don't bother trying to send a message to the RT system if UI Main VI isn't even connected"
          }
          frame True {
            n56 = global read "Global - UI Stream and Variable Connections.vi" "UI Command Stream"() -> (w181:refnum<k21>)
            n57 = shared-variable-write(w181, w184, T18 {"Message"="Send FPGA Configuration to UI", "Message Data"=variant} ("data in")) -> (w183:errorcluster)  [unwired: 1 in, 2 out]
          }
        }
      }
      frame "Initial UI Values" {
        # "Set values of all manual and setpoint controls via reference."
        # "Initial UI Values - These are the current values of the FPGA Main VI's R/W controls. They are used to initialize the panel of UI Main VI upon successful connection to the RT target."
        n58 = Variant To Data(error in=w199, type=T20 {"FPGA State"=enum."Safe State", "Max Acceleration Threshold"=0.0, "Chatter Data"={"Tool data"={"Number of teeth"=2.0}, "Cutting data"={"rpm"=9898.0}, "Limits"={"Magnitude threshold"=0.0, "Tolerance"=1.0}, "G1 status"={"G1 "=FALSE}}}, Variant=w197) -> (data=w196:T20, error out=w198:errorcluster)
        n59 = Unbundle By Name(w195) -> ("Max Acceleration Threshold Ref"=w187:refnum<vi>)
        n60 = Unbundle By Name(w196) -> ("Max Acceleration Threshold"=w189:sgl, "FPGA State"=w188:T5)  [unwired: 1 out]
        n61 = Build Array(w187, w187) -> (w194:refnum<vi>[])
        n62 = Build Array(w189) -> (w193:sgl[])
        n63 = for {
          tunnel: w194 -> [w201] mode=indexing
          tunnel: w193 -> [w200] mode=indexing
          n64 = property class="DigNum (strict)"(reference=w201, "Value"=w200) -> ()  [unwired: 1 in, 2 out]
        }
        n65 = local write "Current FPGA State"(w188) -> ()
        n66 = call "Enqueue Message.vi"("error in (no error)"=w198, "Message Data"=w188, "Message"="Update Display Mode", "Message Queue"=w190) -> ("error out"=w192:errorcluster)  [unwired: 6 in, 1 out]
      }
      frame "Plot and Save" {
        (unwired) u32 1 ("G1?")
        n67 = Variant To Data(error in=w215, type=T21 {"seconds since 1Jan1904"=timestamp(0 s since 1904-01-01), "number"=[], "Machine Data"={"Zload"="", "Yload"="", "Xload"="", "path_position"="", "Fovr"="", "SspeedOvr"="", "Program Name"="", "Program status"="", "Block of code being executed"="", "Line of code"="", "Machine availability"="", "Emergency status"="", "Controller mode"="", "Tool_id"=""}} ("output cluster"), Variant=w214) -> (data=w213:T21, error out=w206:errorcluster)
        n68 = Unbundle(w213) -> ("seconds since 1Jan1904"=w202:timestamp, "number"=w211:dbl[][], "Machine Data"=w209:T24)
        n69 = Index Array(array=w211, index (col)=0 ("disabled index (col)")) -> (element=w207:dbl[])  [unwired: 1 in]
        n70 = call "database_connection_write_dev_MQTT_no_database_array_1.vi"("connection reference"=w203, "string"=w205, "error in (no error)"=w206, "data 2"=w207, "Machine Data"=w209, "current time 2"=w202) -> ("connection reference out"=w204:T16, "error out"=w208:errorcluster)  [unwired: 4 in]
      }
      frame "Plot" {
        (unwired) u32 0 ("G1?")
        (unwired) u32 0 ("G1?")
        n71 = Variant To Data(error in=w230, type=T22 {"seconds since 1Jan1904"=timestamp(0 s since 1904-01-01), "number"=[], "Machine Data"={"Zload"="", "Yload"="", "Xload"="", "path_position"="", "Fovr"="", "SspeedOvr"="", "Program Name"="", "Program status"="", "Block of code being executed"="", "Line of code"="", "Machine availability"="", "Emergency status"="", "Controller mode"="", "Tool id"=""}} ("output cluster"), Variant=w229) -> (data=w227:T22, error out=w220:errorcluster)
        n72 = String To IP() -> ()  [unwired: 1 in, 1 out]
        n73 = Unbundle(w227) -> ("seconds since 1Jan1904"=w221:timestamp, "number"=w225:dbl[][], "Machine Data"=w223:T25)
        n74 = Index Array(array=w225, index (col)=0 ("disabled index (col)")) -> (element=w224:dbl[])  [unwired: 1 in]
        n75 = call "database_connection_write_dev_MQTT_no_database_array_1.vi"("connection reference"=w218, "string"=w219, "error in (no error)"=w220, "data 2"=w224, "Machine Data"=w223, "current time 2"=w221) -> ("connection reference out"=w217:T16, "error out"=w222:errorcluster)  [unwired: 4 in]
      }
      frame "Run Control", "Run Safe State", "Stop Control" {
        # "Run/Stop buttons - Send a command to switch the FPGA into the appropriate state. Send a message to update this UI to reflect the new state."
        n76 = local read "Connected?"() -> (w233:bool)
        n77 = case shown="False" w233 {
          tunnel: w237 -> [w239 w249]
          tunnel: [w239 w245] -> w236
          tunnel: w235 -> [_ w244]
          tunnel: w234 -> [_ w243]
          frame False {
            # "Don't bother trying to send a message to the RT system if UI Main VI isn't even connected"
          }
          frame True {
            # "Run Control switch into Run Control state. Anything else switches to Safe State."
            n78 = case shown="\"Run Control\"" w243 {
              tunnel: [FPGA_State."Safe State" ("FPGA State") FPGA_State."Control (PID)" ("FPGA State")] -> w240
              frame "Safe State", "Stop Control", Default {
              }
              frame "Run Control" {
              }
            }
            n79 = global read "Global - UI Stream and Variable Connections.vi" "UI Command Stream"() -> (w241:refnum<k21>)
            n80 = Bundle("Update FPGA State", "FPGA State"=w240) -> (w246:cluster{string, "FPGA State":T5})  [unwired: 1 in]
            n81 = shared-variable-write(w241, w249, w246) -> (w248:errorcluster)  [unwired: 1 in, 2 out]
            n82 = call "Enqueue Message.vi"("error in (no error)"=w248, "Message Data"=w240, "Message"="Update Display Mode", "Message Queue"=w244) -> ("error out"=w245:errorcluster)  [unwired: 6 in, 1 out]
          }
        }
      }
      frame "Update Control Configuration" {
        # "Update Control Configuration - Send all control configurations to RT to be sent down to the FPGA."
        n83 = Variant To Data(type=T19 {"Tool data"={"Number of teeth"=2.0}, "Cutting data"={"rpm"=9898.0}, "Limits"={"Magnitude threshold"=0.0, "Tolerance"=1.0}, "G1 status"={"G1 "=FALSE}} ("Chatter Data"), Variant=w255) -> (data=w254:T19)  [unwired: 1 in, 1 out]
        n84 = local read "Connected?"() -> (w257:bool)
        n85 = case shown="True" w257 {
          tunnel: w256 -> [w260 w266]
          tunnel: [w260 w265] -> w258
          tunnel: w254 -> [_ w261]
          frame False {
            # "Don't bother trying to send a message to the RT system if UI Main VI isn't even connected"
          }
          frame True {
            n86 = global read "Global - UI Stream and Variable Connections.vi" "UI Command Stream"() -> (w262:refnum<k21>)
            n87 = Bundle("Update Control Configurations", "Chatter Data"=w261) -> (w263:cluster{string, "Chatter Data":T19})  [unwired: 1 in]
            n88 = shared-variable-write(w262, w266, w263) -> (w265:errorcluster)  [unwired: 1 in, 2 out]
          }
        }
      }
      frame "Update Max Acceleration Threshold", "Update Max Fan Speed Threshold", "Update Setpoints" {
        # "Update Manual Values/Setpoints - Send all manual values/setpoints to RT to be sent down to the FPGA."
        n89 = local read "Connected?"() -> (w268:bool)
        n90 = case shown="True" w268 {
          tunnel: [w274 w280] -> w272
          tunnel: w271 -> [w274 w278]
          tunnel: w270 -> [_ w277]
          tunnel: w269 -> [_ w276]
          frame False {
            # "Don't bother trying to send a message to the RT system if UI Main VI isn't even connected"
          }
          frame True {
            n91 = global read "Global - UI Stream and Variable Connections.vi" "UI Command Stream"() -> (w275:refnum<k21>)
            n92 = Bundle(w277, "Message Data"=w276) -> (w279:cluster{string, "Message Data":variant})  [unwired: 1 in]
            n93 = shared-variable-write(w275, w278, w279) -> (w280:errorcluster)  [unwired: 1 in, 2 out]
          }
        }
      }
      frame "Update Display Mode" {
        # "Update Display Mode - Enable/Disable Controls appropriately for the new display mode."
        n94 = Variant To Data(error in=w290, type=FPGA_State."Safe State" ("FPGA State"), Variant=w288) -> (data=w286:T5, error out=w289:errorcluster)
        n95 = Unbundle By Name(w287) -> ("Switch to Safe State Ref"=w285:refnum<vi>, "Stop Control Ref"=w283:refnum<vi>, "Run Control Ref"=w282:refnum<vi>)
        n96 = case shown="\"Control (PID)\"" w286 {
          tunnel: w285 -> [w293 w299]
          tunnel: w282 -> [w291 w300]
          tunnel: w283 -> [w292 w298]
          frame "Control (PID)" {
            n97 = Build Array "Controls to Enable"(w293, w292) -> (w297:refnum<vi>[])
            n98 = Build Array "Controls to Disable"(w291) -> (w295:refnum<vi>[])
            n99 = call "Set Enable State on Multiple Controls.vi"("Enable?"=FALSE, "Controls"=w295) -> ()  [unwired: 10 in]
            n100 = call "Set Enable State on Multiple Controls.vi"("Enable?"=TRUE, "Controls"=w297) -> ()  [unwired: 10 in]
          }
          frame "Safe State", Default {
            # "This frame runs when FPGA is in Safe State. Only enable the run button."
            n101 = Build Array "Controls to Enable"(w300) -> (w304:refnum<vi>[])
            n102 = Build Array "Controls to Disable"(w299, w298) -> (w302:refnum<vi>[])
            n103 = call "Set Enable State on Multiple Controls.vi"("Enable?"=FALSE, "Controls"=w302) -> ()  [unwired: 10 in]
            n104 = call "Set Enable State on Multiple Controls.vi"("Enable?"=TRUE, "Controls"=w304) -> ()  [unwired: 10 in]
          }
        }
      }
      frame "Critical Error", "Log-Only Error", "Non-Critical Error", "RT Error" {
        # "Error - Display message in status indicator on panel.  If it's a critical error, shut down this VI with an 'Exit' message."
        n105 = case shown="Default" w307 {
          selector: w307 -> [_ w325]
          tunnel: ["UI Error" w325] -> w306
          frame Default {
          }
          frame "RT Error" {
          }
        }
        n106 = Variant To Data(error in=w321, type=errorcluster {"status"=FALSE, "code"=0, "source"=""} ("error constant"), Variant=w319) -> (data=w314:errorcluster, error out=w320:errorcluster)
        n107 = Unbundle By Name(w314) -> ("code"=w313:i32, "source"=w317:string)
        n108 = Format Date/Time String() -> (date/time string=w316:string)  [unwired: 3 in]
        n109 = Format Into String(format string="\n%s: %s %d - %s", w316, w306, w313, w317) -> (resulting string=w308:string)  [unwired: 2 in, 1 out]
        n110 = call "Enqueue Message.vi"("error in (no error)"=w320, "Message Data"=w308, "Message"="Update System Status", "Message Queue"=w311) -> ("error out"=w312:errorcluster, "dup Message Queue"=w310:refnum<queue>)  [unwired: 6 in]
        n111 = case shown="Default" w307 {
          tunnel: w312 -> [w326 w330]
          tunnel: w310 -> [_ w328]
          tunnel: [w326 w329] -> w322
          frame Default {
          }
          frame "Critical Error" {
            n112 = call "Enqueue Message.vi"("error in (no error)"=w330, "Message"="Exit", "Message Queue"=w328) -> ("error out"=w329:errorcluster)  [unwired: 7 in, 1 out]
          }
        }
      }
      frame "Update System Status" {
        # "#CodeRecommended - The code below ensures that the System Status string value does not become too large.  It uses the same maximum size as the RT error log to determine whether or not to remove the last half of the log string. Change this logic if you wish to maintain more/less of the information in the System Status string."
        # "Update System Status - Add a new string to the beginning of the System Status string on the UI."
        n113 = Variant To Data(error in=w343, type="", Variant=w340) -> (data=w337:string, error out=w341:errorcluster)
        n114 = local read "System Status"() -> (w335:string)
        n115 = global read "Global - Configuration Options.vi" "Error Log Max Size (bytes)"() -> (w333:i64)
        n116 = String Length(string=w335) -> (length=w336:i32)
        n117 = Greater?(x=w336, y=w333) -> (0:w334:bool)
        n118 = case shown="False" w334 {
          tunnel: w335 -> [w344 w348]
          tunnel: w333 -> [_ w347]
          tunnel: [w344 w349] -> w332
          frame False {
          }
          frame True {
            n119 = Divide(x=w347, y=i64 2) -> (x/y=w346:dbl)
            n120 = String Subset(string=w348, length (rest)=w346) -> (substring=w349:string)  [unwired: 1 in]
          }
        }
        n121 = Concatenate Strings(w337, w332) -> (→"System Status":string)
      }
      frame "Exit" {
        # "Close all connections"
        # "Stop Monitoring Loop"
        # "Stop Event Handling Loop"
        # "Release the UI Message queue reference"
        # "Stop UI Message Loop"
        # "Exit - Fire the User Event to stop the Event Handling Loop, and toggle the local variable to stop the Monitoring Loop.  This message alone causes all three loops to stop."
        n122 = local write "Connected?"(FALSE ("Connected?")) -> ()
        n123 = global write "Global - All UI Loop Stop.vi" "All UI Loop Stop"(TRUE ("Stop Monitoring Loop")) -> ()
        n124 = call "Fire User Event - Stop.vi"("User Event - Stop"=w360) -> ("error out"=w359:errorcluster)  [unwired: 10 in]
        n125 = Release Queue(queue=w356, error in (no error)=w361) -> (error out=w357:errorcluster)  [unwired: 1 in, 2 out]
        n126 = global read "Global - UI Stream and Variable Connections.vi" "UI Command Stream"() -> (w355:refnum<k21>)
        n127 = global read "Global - UI Stream and Variable Connections.vi" "RT Message Stream"() -> (w354:refnum<k21>)
        n128 = global read "Global - UI Stream and Variable Connections.vi" "Variable References"() -> (w351:T23)
        n129 = Destroy Stream Endpoint(11:w355) -> ()  [unwired: 1 in, 1 out]
        n130 = Destroy Stream Endpoint(11:w354) -> ()  [unwired: 1 in, 1 out]
        n131 = Merge Errors(w359, w357) -> (w362:errorcluster)
        n132 = call "Close Variable Connections.vi"("Variable References 2"=w351) -> ()  [unwired: 11 in]
      }
      frame "---Copy This Frame---" {
        # "Duplicate this frame when creating new messages.  Change this comment in the duplicated frame to describe this message."
        n133 = Merge Errors(w367) -> (w366:errorcluster)
      }
      frame "Update Tool Data" {
        # "Duplicate this frame when creating new messages.  Change this comment in the duplicated frame to describe this message."
        n134 = Variant To Data(type=path "" ("Tool Data File"), Variant=w377) -> (data=w369:path, error out=w371:errorcluster)  [unwired: 1 in]
        n135 = Build Path(name or relative path=w369) -> (appended path=w375:path)  [unwired: 1 in]
        n136 = Read from Text File(file (use dialog)=w375, error in=w371) -> (text=w372:string, error out=w374:errorcluster)  [unwired: 2 in, 2 out]
        n137 = Unbundle By Name(w374) -> ("status"=w373:bool)  [unwired: 1 out]
        n138 = case shown="False" w373 {
          tunnel: w372 -> [w381 _]
          tunnel: [w381 "Error"] -> w370
          frame False {
          }
          frame True {
          }
        }
        "Tool Data" <- w370
        n139 = Merge Errors(w380) -> (w379:errorcluster)
      }
      frame "Unsuccessful Connection" {
        # "Duplicate this frame when creating new messages.  Change this comment in the duplicated frame to describe this message."
        n140 = flat-sequence {
          tunnel: w388 -> [w391]
          tunnel: [w391] -> w387
          tunnel: w387 -> [w392]
          tunnel: w386 -> [w405]
          tunnel: [w404] -> w384
          tunnel: w385 -> [w403]
          frame #0 {
            n141 = local write "Connected?"(FALSE ("Connected?")) -> ()
          }
          frame #1 {
            w393 = 0
            n142 = Unbundle(w392) -> ("Switch to Safe State Ref"=w401:refnum<vi>, "Run Control Ref"=w400:refnum<vi>, "Stop Control Ref"=w399:refnum<vi>, "Update Control Configurations Ref"=w398:refnum<vi>, "Chatter Data Ref"=w397:refnum<vi>, "Max Acceleration Threshold Ref"=w396:refnum<vi>)
            n143 = property on="Controller Address" class="Str"("DisabledEnum"=w393) -> ()  [unwired: 2 in, 2 out]
            n144 = property on="Connect to Controller" class="Bool"("DisabledEnum"=w393) -> ()  [unwired: 2 in, 2 out]
            n145 = Build Array(w401, w400, w399, w398, w397, w396) -> (w395:refnum<vi>[])
            n146 = call "Set Enable State on Multiple Controls.vi"("Enable?"=FALSE, "Controls"=w395) -> ()  [unwired: 10 in]
          }
          frame #2 {
            n147 = Wait (ms)(milliseconds to wait=u32 1000) -> ()  [unwired: 1 out]
          }
          frame #3 {
            n148 = call "Enqueue Message.vi"("error in (no error)"=w405, "Message"="Connect", "Message Queue"=w403) -> ("error out"=w404:errorcluster)  [unwired: 7 in, 1 out]
          }
        }
        n149 = Merge Errors(w384) -> (w389:errorcluster)
      }
      frame Default {
        # "'Default' case only runs if there is a message that isn't defined in any of the other cases.  Output a programming error."
        n150 = Format Into String(format string="The invalid message string \"%s\" was received in the Message Handling Loop." ("Invalid Message Loop Message"), w412) -> (resulting string=w409:string)  [unwired: 2 in, 1 out]
        n151 = call <vilib>:"Error Cluster From Error Code.vi"("error message (\"\")"=w409, "error code (0)"=1) -> ("error out"=w410:errorcluster)  [unwired: 7 in]
      }
    }
    n152 = call "UI Error Handler - Message Handler.vi"("error in (no error)"=w69, "Message Queue"=w70) -> ()  [unwired: 9 in, 1 out]
    n153 = call <vilib>:"Clear Errors.vi"("error in (no error)"=w69) -> ("error out"=w68:errorcluster)  [unwired: 5 in, 1 out]
  }
  n154 = Tick Count (ms)() -> (millisecond timer value=w35:u32)
  n155 = while {
    tunnel: w47 -> [w414]
    tunnel: [w417] -> w57
    shift-right: [w415] -> w49
    shift-left: w55 -> [w416]
    stop <- w418 stop-if-true
    # "Event Handling Loop"
    n156 = event shown="[0] \"Connect to Controller\": Value Change" {
      selector: w416 -> [_ _ _ _ _ _ _ _]
      dyn-events: [_ _ _ _ _ _ _ _] -> w415
      timeout: _ -> [_ _ _ _ _ _ _ _]
      tunnel: [_ _ _ _ _ _ _ TRUE ("Discard?")] -> w419
      tunnel: w414 -> [w425 w428 w431 w434 w439 _ w444 _]
      tunnel: [w427 w430 w433 w436 w438 _ w447 _] -> w417
      tunnel: w414 -> [_ _ _ _ _ w443 _ _]
      event "Connect to Controller": Value Change {
        n157 = event-data() -> ()  [unwired: 1 in, 1 out]
        n158 = call "Enqueue Message.vi"("Message"="Connect", "Message Queue"=w425) -> ("error out"=w427:errorcluster)  [unwired: 8 in, 1 out]
      }
      event "Run Control": Value Change {
        n159 = event-data() -> ()  [unwired: 1 in, 1 out]
        n160 = call "Enqueue Message.vi"("Message"="Run Control", "Message Queue"=w428) -> ("error out"=w430:errorcluster)  [unwired: 8 in, 1 out]
      }
      event "Stop Control": Value Change {
        n161 = event-data() -> ()  [unwired: 1 in, 1 out]
        n162 = call "Enqueue Message.vi"("Message"="Stop Control", "Message Queue"=w431) -> ("error out"=w433:errorcluster)  [unwired: 8 in, 1 out]
      }
      event "Switch to Safe State": Value Change {
        n163 = event-data() -> ()  [unwired: 1 in, 1 out]
        n164 = call "Enqueue Message.vi"("Message"="Run Safe State", "Message Queue"=w434) -> ("error out"=w436:errorcluster)  [unwired: 8 in, 1 out]
      }
      event "Max Acceleration Threshold (g)": Value Change {
        n165 = event-data() -> ()  [unwired: 1 in, 1 out]
        n166 = call "Enqueue Message.vi"("Message Data"="Max Acceleration Threshold (g)", "Message"="Update Max Acceleration Threshold", "Message Queue"=w439) -> ("error out"=w438:errorcluster)  [unwired: 7 in, 1 out]
      }
      event "Tool Data File", "OK Button": Value Change {
        n167 = event-data() -> ()  [unwired: 1 in, 3 out]
        n168 = call "Enqueue Message.vi"("Message Data"="Tool Data File", "Message"="Update Tool Data", "Message Queue"=w443) -> ()  [unwired: 7 in, 2 out]
      }
      event "Exit": Value Change {
        w445 = TRUE  # Priority Message
        # "The UI Message Loop handles sending the Exit message to other loops."
        n169 = event-data() -> ()  [unwired: 1 in, 1 out]
        n170 = call "Enqueue Message.vi"("Priority Message? (F)"=w445, "Message"="Exit", "Message Queue"=w444) -> ("error out"=w447:errorcluster)  [unwired: 7 in, 1 out]
      }
      event User Event {
        # "The Message Handling Loop processed an \"Exit\" message, which fired this event to stop the Event Handling Loop."
        n171 = event-data() -> ()  [unwired: 1 in, 1 out]
      }
    }
    n172 = case shown="Error" w417 {
      tunnel: [w420 TRUE ("Discard?")] -> w418
      tunnel: w419 -> [w420 _]
      tunnel: w414 -> [_ w421]
      frame No Error {
      }
      frame Error {
        # "On error, send Exit message, and stop loop."
        n173 = call "Enqueue Message.vi"("Priority Message? (F)"=TRUE ("Discard?"), "Message"="Exit", "Message Queue"=w421) -> ()  [unwired: 7 in, 2 out]
      }
    }
  }
  n174 = call "mqttTXdataQueue.vi"("function"=mqttTXdataQueueFunction."init", "error in (no error)"="error in (no error)") -> ("error out"=w5:errorcluster)  [unwired: 12 in, 1 out]
  n175 = call "api_mqttInit.vi"("client"=w8, "broker"=T9 {"address"="localhost", "port"=1883, "connTimeout"=2000, "writeTimeout"=2000, "readTimeout"=2000, "subTimeout"=30000}, "connFlags"=T11 {"reserved"=FALSE, "clean session"=TRUE, "will flag"=TRUE, "willQOS"=enum."At most once", "will retain"=FALSE, "password"=FALSE, "user name"=FALSE}, "User Info"=T10 {"User Name"="User", "Password"="password"}, "error in (no error)"=w5) -> ("error out"=w6:errorcluster)  [unwired: 10 in]
  n176 = call "mqttConfigStore.vi"("function"=mqttConfigFunction."get", "error in (no error)"=w6) -> ("mqtt.lvclass out"=w13:refnum<class "mqtt.lvclass">, "error out"=w12:errorcluster)  [unwired: 12 in]
  n177 = call "mqttTCPIPserver.vi"("mqtt.lvclass"=w13, "error in (no error)"=w12) -> ()  [unwired: 12 in, 2 out]
  n178 = call "api_mqttConnect.vi"("error in (no error)"=w12) -> ("success"=→"success":bool, "connStatus"=→"connStatus 2":T3, "sessionPresent"=→"sessionPresent 2":bool, "error out"=w4:errorcluster)  [unwired: 11 in]
  n179 = while {
    tunnel: w47 -> [w454]
    tunnel: "milliseconds to wait" -> [w459]
    shift-right: [w455] -> _
    shift-left: w39 -> [w456]
    tunnel: w36 -> [w458]
    tunnel: w40 -> [w457]
    shift-right: [w451] -> _
    shift-left: w35 -> [w453]
    shift-right: [w449] -> _
    shift-left: w4 -> [w450]
    stop <- w461 stop-if-true
    # "Only read monitoring variables if the UI Main VI is connected to the RT target"
    # "Only the 'Exit' message in the UI Message Loop can stop the Monitoring Loop."
    # "Monitoring Loop"
    n180 = Tick Count (ms)() -> (millisecond timer value=w451:u32)
    n181 = Subtract(x=w451, y=w453) -> (x-y=→"Loop execution":u32)
    n182 = local read "Connected?"() -> (w460:bool)
    n183 = case shown="True" w460 {
      tunnel: w454 -> [_ w601]
      tunnel: w459 -> [w464 w597]
      tunnel: w456 -> [_ w585]
      tunnel: w458 -> [_ w584]
      tunnel: w457 -> [_ w583]
      tunnel: [w463 w582] -> w455
      tunnel: w456 -> [w463 w582]
      tunnel: w454 -> [_ w581]
      tunnel: w450 -> [w462 _]
      tunnel: w450 -> [_ w473]
      tunnel: [w462 w474] -> w449
      frame False {
        n184 = Wait (ms)(milliseconds to wait=w464) -> ()  [unwired: 1 out]
      }
      frame True {
        (unwired) 1 ("length")
        (unwired) sgl 0.0 ("Tolerance")
        # "Serialize the shared variable calls to simplify the scheduling performed by LabVIEW at runtime"
        n185 = Unbundle By Name("connMeta") -> ("qos"=w484:T2, "retain"=w483:bool, "duplicate"=w482:bool)
        n186 = feedback #1(u16 0) -> (w489:u16)
        n187 = Increment(x=w489) -> (x+1=w488:u16)
        "publishMessageID" <- w488
        n188 = feedback-in #1(w488) -> ()
        n189 = global read "Global - UI Stream and Variable Connections.vi" "Variable References"() -> (w599:T23)
        n190 = Unbundle By Name(w599) -> ("Current FPGA State"=w596:refnum<k21>, "Acceleration (grms)"=w593:refnum<k21>, "Acceleration Waveform"=w592:refnum<k21>, "Chatter"=w525:refnum<k21>, "tag acc"=w531:refnum<k21>, "tag video"=w530:refnum<k21>, "Free or Contiguous Memory"=w498:refnum<k21>, "DMA FIFO Overflow?"=w511:refnum<k21>, "CPU Usage"=w510:refnum<k21>, "Image Waveform"=w495:refnum<k21>)
        n191 = call "UI - Read Stream from RT.vi"("Message Queue"=w601) -> ("Message Received?"=w598:bool, "dup Message Queue"=w600:refnum<queue>)  [unwired: 8 in, 1 out]
        n192 = case shown="False" w598 {
          tunnel: w597 -> [w755 _]
          frame False {
            n193 = Wait Until Next ms Multiple(millisecond multiple=w755) -> ()  [unwired: 1 out]
          }
          frame True {
            # "If a message was received, immediately read again"
          }
        }
        n194 = shared-variable-read(w495) -> (w494:T28[])  [unwired: 1 in, 3 out]
        n195 = shared-variable-read(w596) -> (w595:errorcluster, w587:T27)  [unwired: 1 in, 2 out]
        "Current FPGA State" <- w587
        n196 = shared-variable-read(w593, w595) -> (w594:errorcluster, w466:dbl[])  [unwired: 2 out]
        n197 = shared-variable-read(w592, w594) -> (w575:errorcluster, w469:waveform(dbl)[], w500:timestamp)  [unwired: 1 out]
        n198 = shared-variable-read(w525, w575) -> (w532:errorcluster, w574:bool[])  [unwired: 2 out]
        n199 = shared-variable-read(w531, w532) -> (w529:errorcluster, w493:string)  [unwired: 2 out]
        "tag acc" <- w493
        "string" <- w493
        n200 = shared-variable-read(w530, w529) -> (w528:errorcluster, w497:string)  [unwired: 2 out]
        "tag spike" <- w497
        n201 = Boolean To (0,1)(Boolean=w574) -> (0, 1=w519:i16[])
        n202 = for {
          tunnel: w585 -> [w630] mode=indexing
          shift-right: [w632] -> w580
          shift-left: w528 -> [w631]
          tunnel: [w624] -> w558 mode=indexing
          tunnel: [w629] -> w572
          tunnel: w581 -> [w629]
          tunnel: w583 -> [w628]
          tunnel: w584 -> [w627]
          tunnel: [w625] -> w527
          tunnel: [w626] -> w522
          n203 = case "Message Cases" shown="\"Machine Data\"" w630 {
            tunnel: w631 -> [_ _ _ w651 w659 w666 w673 w680 w687 w694 w701 w708 w715 w722 w729 w736 _]
            tunnel: [_ _ _ _ w659 w666 w673 w680 w687 w694 w701 w708 w715 w722 w729 w736 _] -> w632
            tunnel: [w633 w640 w643 w646 w654 w661 w668 w675 w682 w689 w697 w703 w711 w717 w724 w733 w737] -> w624
            tunnel: w628 -> [w635 w639 w645 w650 w655 w662 w669 w676 w683 w690 w695 w707 w709 w721 w725 w731 _]
            tunnel: w627 -> [_ _ _ _ _ _ _ _ _ _ _ _ _ _ _ _ w739]
            tunnel: [FALSE ("Triggger G1,G2, or G3") FALSE ("Triggger G1,G2, or G3") FALSE ("Triggger G1,G2, or G3") FALSE ("Triggger G1,G2, or G3") FALSE ("Triggger G1,G2, or G3") FALSE ("Triggger G1,G2, or G3") FALSE ("Triggger G1,G2, or G3") FALSE ("Triggger G1,G2, or G3") FALSE ("Triggger G1,G2, or G3") FALSE ("Triggger G1,G2, or G3") FALSE ("Triggger G1,G2, or G3") FALSE ("Triggger G1,G2, or G3") FALSE ("Triggger G1,G2, or G3") FALSE ("Triggger G1,G2, or G3") FALSE ("Triggger G1,G2, or G3") FALSE ("Triggger G1,G2, or G3") w744] -> w625
            tunnel: [_ _ _ _ _ _ _ _ _ _ _ _ _ _ _ _ w738] -> w626
            frame "Spindle Load" {
              # "maximum spindle power"
              # "Action 1 - Send an \"Update Display\" message indicating which button was pressed. Note that a string is sent as the Message Data along with the \"Update Display\" message."
              n204 = call "read_data_spindle_load_mt_connect (SubVI).vi"("URL"=w635) -> ("number"=w636:dbl[])  [unwired: 9 in, 1 out]
              n205 = Multiply(x=1, y=w636) -> (x*y=w633:dbl[])
              "Spindle Load" <- w633
            }
            frame "Spindle Speed" {
              # "Action 2 - Send an \"Update Display\" message indicating which button was pressed. Note that a string is sent as the Message Data along with the \"Update Display\" message."
              n206 = call "read_data_speed_mt_connect (SubVI).vi"("URL"=w639) -> ("number"=w640:dbl[])  [unwired: 9 in, 1 out]
            }
            frame "Feed Rate", Default {
              n207 = call "read_data_feed_mt_connect (SubVI).vi"("URL"=w645) -> ("appended array"=w643:dbl[])  [unwired: 9 in, 1 out]
              n208 = Index Array(array=w643, index=0) -> (element=→"Feed":dbl)
            }
            frame "Position I" {
              n209 = call "read_data_linear_position_mt_connect (SubVI).vi"("error in (no error)"=w651, "URL"=w650) -> ("I, J,K,X, Y,Z"=w648:dbl[])  [unwired: 8 in, 1 out]
              n210 = Index Array(array=w648, index=0) -> (element=w647:dbl)
              n211 = Build Array(w647) -> (w646:dbl[])
            }
            frame "Position J" {
              n212 = call "read_data_linear_position_mt_connect (SubVI).vi"("URL"=w655) -> ("I, J,K,X, Y,Z"=w657:dbl[])  [unwired: 9 in, 1 out]
              n213 = Index Array(array=w657, index=1) -> (element=w656:dbl)
              n214 = Build Array(w656) -> (w654:dbl[])
            }
            frame "Position K" {
              n215 = call "read_data_linear_position_mt_connect (SubVI).vi"("URL"=w662) -> ("I, J,K,X, Y,Z"=w664:dbl[])  [unwired: 9 in, 1 out]
              n216 = Index Array(array=w664, index=2) -> (element=w663:dbl)
              n217 = Build Array(w663) -> (w661:dbl[])
            }
            frame "Position X" {
              n218 = call "read_data_linear_position_mt_connect (SubVI).vi"("URL"=w669) -> ("I, J,K,X, Y,Z"=w671:dbl[])  [unwired: 9 in, 1 out]
              n219 = Index Array(array=w671, index=3) -> (element=w670:dbl)
              n220 = Build Array(w670) -> (w668:dbl[])
            }
            frame "Position Y" {
              n221 = call "read_data_linear_position_mt_connect (SubVI).vi"("URL"=w676) -> ("I, J,K,X, Y,Z"=w678:dbl[])  [unwired: 9 in, 1 out]
              n222 = Index Array(array=w678, index=4) -> (element=w677:dbl)
              n223 = Build Array(w677) -> (w675:dbl[])
            }
            frame "Position Z" {
              n224 = call "read_data_linear_position_mt_connect (SubVI).vi"("URL"=w683) -> ("I, J,K,X, Y,Z"=w685:dbl[])  [unwired: 9 in, 1 out]
              n225 = Index Array(array=w685, index=5) -> (element=w684:dbl)
              n226 = Build Array(w684) -> (w682:dbl[])
            }
            frame "Position A" {
              n227 = call "read_data_linear_angle_mt_connect (SubVI).vi"("URL"=w690) -> ("I, J,K,X, Y,Z"=w692:dbl[])  [unwired: 9 in, 1 out]
              n228 = Index Array(array=w692, index=0) -> (element=w691:dbl)
              n229 = Build Array(w691) -> (w689:dbl[])
            }
            frame "Position B" {
              n230 = call "read_data_linear_angle_mt_connect (SubVI).vi"("URL"=w695) -> ("I, J,K,X, Y,Z"=w699:dbl[])  [unwired: 9 in, 1 out]
              n231 = Index Array(array=w699, index=1) -> (element=w698:dbl)
              n232 = Build Array(w698) -> (w697:dbl[])
            }
            frame "Xload" {
              n233 = call "read_data_linear_loadX_mt_connect (SubVI).vi"("URL"=w707) -> ("I, J,K,X, Y,Z"=w705:dbl[])  [unwired: 9 in, 1 out]
              n234 = Index Array(array=w705, index=0) -> (element=w704:dbl)
              n235 = Build Array(w704) -> (w703:dbl[])
            }
            frame "Yload" {
              n236 = call "read_data_linear_loadX_mt_connect (SubVI).vi"("URL"=w709) -> ("I, J,K,X, Y,Z"=w713:dbl[])  [unwired: 9 in, 1 out]
              n237 = Index Array(array=w713, index=1) -> (element=w712:dbl)
              n238 = Build Array(w712) -> (w711:dbl[])
            }
            frame "Zload" {
              n239 = call "read_data_linear_loadX_mt_connect (SubVI).vi"("URL"=w721) -> ("I, J,K,X, Y,Z"=w718:dbl[])  [unwired: 9 in, 1 out]
              n240 = Index Array(array=w718, index=2) -> (element=w719:dbl)
              n241 = Build Array(w719) -> (w717:dbl[])
            }
            frame "Aload" {
              n242 = call "read_data_angle_loadmt_connect (SubVI).vi"("URL"=w725) -> ("I, J,K,X, Y,Z"=w727:dbl[])  [unwired: 9 in, 1 out]
              n243 = Index Array(array=w727, index=0) -> (element=w726:dbl)
              n244 = Build Array(w726) -> (w724:dbl[])
            }
            frame "Bload" {
              n245 = call "read_data_angle_loadmt_connect (SubVI).vi"("URL"=w731) -> ("I, J,K,X, Y,Z"=w730:dbl[])  [unwired: 9 in, 1 out]
              n246 = Index Array(array=w730, index=1) -> (element=w735:dbl)
              n247 = Build Array(w735) -> (w733:dbl[])
            }
            frame "Machine Data" {
              n248 = call "read_machine_parameters_mt_connect (SubVI).vi"("URL 2"=w739) -> ("Machine Data"=w738:T24)  [unwired: 8 in, 1 out]
              n249 = Unbundle By Name(w738) -> ("Block of code being executed"=w745:string)
              "Block of code being executed" <- w745
              n250 = Unbundle By Name(w738) -> ("Tool_id"=→"Tool id":string, "Program Name"=w743:string)
              "Program Name" <- w743
              n251 = Decimal String To Number(string=w743) -> (number=w742:i32)  [unwired: 2 in, 1 out]
              n252 = call "check_G1_G2_G3.vi"("current line"=w745) -> ("Triggger G1,G2, or G3"=w744:bool)  [unwired: 8 in, 1 out]
              n253 = To Double Precision Float(number=w742) -> (double precision float=w741:dbl)
              n254 = Build Array(w741) -> (w737:dbl[])
            }
          }
        }
        n255 = Or(x=w527, y="Save?") -> (x .or. y?=w504:bool)
        n256 = Equal?(x=w587, y=FPGA_state."Safe State") -> (x = y?=w589:bool)
        n257 = feedback #2(timestamp(0 s since 1904-01-01)) -> (w591:timestamp)
        n258 = feedback-in #2(w500) -> ()
        n259 = case shown="True" w589 {
          frame False {
            n260 = property on="Run Control" class="Bool"("DisabledEnum"=T13."Disabled and Grayed Out" ("Disabled")) -> ()  [unwired: 2 in, 2 out]
            n261 = property on="Stop Control" class="Bool"("DisabledEnum"=T13."Enabled" ("Disabled")) -> ()  [unwired: 2 in, 2 out]
          }
          frame True {
            n262 = property on="Run Control" class="Bool"("DisabledEnum"=T13."Enabled" ("Disabled")) -> ()  [unwired: 2 in, 2 out]
            n263 = property on="Stop Control" class="Bool"("DisabledEnum"=T13."Disabled and Grayed Out" ("Disabled")) -> ()  [unwired: 2 in, 2 out]
          }
        }
        n264 = Array Subset(array=w466, index=0, length=11) -> (w491:dbl[])
        n265 = Equal?(x=w500, y=w591) -> (x = y?=w526:bool)
        n266 = Array To Cluster(array=w491) -> (cluster=→"ACC  (grms)":T7)
        n267 = control-ref of="H5 machine"() -> (w551:refnum<vi>)
        n268 = shared-variable-read(w498) -> (→"Free Physical Memory or Largest Contiguous Memory (bytes)":dbl)  [unwired: 1 in, 3 out]
        n269 = case shown="False" w526 {
          tunnel: w469 -> [_ w754]
          tunnel: w469 -> [w751 _]
          tunnel: [w751 w754] -> w499
          frame False {
            n270 = Array Subset(array=w751, index=0, length=11) -> (→"Raw ACC":waveform(dbl)[])
            "Raw Waveform 2" <- w751
          }
          frame True {
          }
        }
        n271 = property on="Property Node" class="Bool (strict)"(reference=w551) -> ("Colors [4]"=w545:cluster{u32, u32}[])  [unwired: 1 in, 2 out]
        n272 = shared-variable-read(w511) -> (w517:errorcluster, →"DMA FIFO Overflow?":bool)  [unwired: 1 in, 2 out]
        n273 = shared-variable-read(w510, w517) -> (w516:T29)  [unwired: 3 out]
        n274 = Array Size(array=w466) -> (size(s)=→"size(s) 2":i32)
        n275 = for {
          tunnel: w516 -> [w607] mode=indexing
          tunnel: [w606] -> w515 mode=indexing
          n276 = Unbundle By Name(w607) -> ("Total (%)"=w606:dbl)
        }
        n277 = Bundle By Name(cluster=T26 {"Magnitude threshold"=0.0, "Tolerance"=0.0} ("Limits"), "Magnitude threshold"=sgl 0.00015, "Tolerance"=sgl 2.0) -> (w564:T26)
        n278 = Array Size(array=w515) -> (size(s)=w514:i32)
        n279 = Reshape Array(w515, 1 ("dimension size"), w514) -> (→"CPU Usage (%)":dbl[][])
        n280 = Index Array(array=w545, index=2) -> (element=w547:cluster{u32, u32})
        n281 = Array Subset(array=w466, index=15, length=6) -> (w534:dbl[])
        n282 = Array Subset(array=w466, index=11, length=4) -> (w468:dbl[])
        n283 = Array To Cluster(array=w468) -> (cluster=→"Automated FRF  (grms) 2":T6)
        n284 = Array Size(array=w468) -> (size(s)=→"size(s)":i32)
        n285 = Get Date/Time In Seconds() -> (seconds since 1Jan1904=w586:timestamp)
        n286 = Index Array(array=w558, index (row)=1, index (col)=0 ("disabled index (col)")) -> (element=w559:dbl)
        "RPM" <- w559
        n287 = Bundle By Name(cluster=cluster{"rpm":sgl} {"rpm"=0.0} ("Cutting data"), "rpm"=w559) -> (w566:cluster{"rpm":sgl})
        n288 = Build Array(w491) -> (w577:dbl[][])
        n289 = Array To Cluster(array=w534) -> (cluster=→"Strain (grms)":T8)
        n290 = Transpose 2D Array(2D array=w577) -> (transposed array=w576:dbl[][])
        n291 = Or(x="Save?", y=w527) -> (x .or. y?=w524:bool)
        n292 = Insert Into Array(array=w558, new element=w576) -> (w492:dbl[][])  [unwired: 2 in]
        n293 = case shown="False" w524 {
          tunnel: w493 -> [_ w612]
          tunnel: [w610 w614] -> w523
          tunnel: w522 -> [w611 w613]
          tunnel: w497 -> [_ _]
          frame False {
            n294 = Bundle By Name(cluster=w611, "path_position"="Unavailable" ("Tool_id"), "Xload"="Unavailable" ("Tool_id")) -> (w610:T24)
          }
          frame True {
            n295 = Bundle By Name(cluster=w613, "path_position"=w612, "Xload"=w612) -> (w614:T24)
          }
        }
        n296 = Bundle("seconds since 1Jan1904"=w586, "appended array"=w492, "Machine Data"=w523) -> (w475:T30)  [unwired: 1 in]
        n297 = Unbundle(w475) -> ("seconds since 1Jan1904"=w481:timestamp, "appended array"=w479:dbl[][], "Machine Data"=w480:T24)
        n298 = Index Array(array=w479, index (col)=0 ("disabled index (col)")) -> (element=w477:dbl[])  [unwired: 1 in]
        n299 = call "MQTT_10Hz.vi"("data 2"=w477, "Machine Data"=w480, "current time 2"=w481) -> ("JSON string"=w476:string)  [unwired: 8 in]
        n300 = call "api_mqttPublish.vi"("topic"="topic", "value"=w476, "QoS (At most once)"=w484, "messageID"=w488, "error in (no error)"=w473, "retain(F)"=w483, "duplicate(F)"=w482) -> ("success"=→"publishSuccess":bool, "error out"=w474:errorcluster)  [unwired: 7 in]
        n301 = To Variant(anything=w475) -> (Variant=w578:variant)
        n302 = Unbundle By Name(w522) -> ("Program status"=w507:string)
        n303 = case shown="\"INTERRUPTED\"" w507 {
          tunnel: [u32 16723242 u32 6618880 u32 16449369 u32 16449369 u32 16449369] -> w544
          frame "Stopped", Default {
          }
          frame "ACTIVE" {
          }
          frame "INTERRUPTED" {
          }
          frame "FEED_HOLD" {
          }
          frame "READY" {
          }
        }
        n304 = Bundle(cluster=w547, w544) -> (w548:cluster{u32, u32})  [unwired: 1 in]
        n305 = Insert Into Array(array=w545, index=0, new element #1=w548, new element #2=w548, new element #3=w548, new element #4=w548) -> (w546:cluster{u32, u32}[])
        n306 = property on="Property Node" class="Bool (strict)"(reference=w551, "Colors [4]"=w546) -> ()  [unwired: 1 in, 2 out]
        n307 = Equal?(x=w507, y="ACTIVE") -> (x = y?=w506:bool)
        n308 = Index Array(array=w558, index (row)=0, index (col)=0 ("disabled index (col)")) -> (element=w555:dbl)
        n309 = Greater?(x=w555, y="In-cut Power Threshold") -> (0:w540:bool)
        n310 = And(x=w540, y=w524) -> (x .and. y?=w539:bool)
        n311 = case shown="False" w539 {
          tunnel: w519 -> [_ w621]
          tunnel: [w620 w621] -> w543
          tunnel: i16[] [0, 0, 0] ("0, 1") -> [w620 _]
          frame False {
          }
          frame True {
          }
        }
        n312 = Not Equal To 0?(x=w543) -> (x != 0?=w542:bool[])
        n313 = Or Array Elements(Boolean array=w542) -> (logical OR=→"Chatter?":bool)
        n314 = case shown="True" w506 {
          tunnel: [sgl 0.0 ("Tolerance") sgl 1.0 ("Tolerance")] -> w505
          tunnel: [FALSE TRUE] -> w503
          frame False {
          }
          frame True {
          }
        }
        n315 = Or(x=w504, y=w503) -> (x .or. y?=w502:bool)
        "x .or. y?" <- w502
        n316 = Bundle By Name(cluster=cluster{"Number of teeth":sgl} {"Number of teeth"=0.0} ("Tool data"), "Number of teeth"=w505) -> (w568:cluster{"Number of teeth":sgl})
        n317 = Bundle By Name(cluster=cluster{"G1 ":bool} {"G1 "=FALSE} ("G1 status"), "G1"=w502) -> (w496:cluster{"G1 ":bool})
        "output cluster" <- w496
        n318 = Bundle By Name(cluster=T19 {"Tool data"={"Number of teeth"=2.0}, "Cutting data"={"rpm"=9898.0}, "Limits"={"Magnitude threshold"=0.0, "Tolerance"=1.0}, "G1 status"={"G1 "=FALSE}} ("Chatter Data"), "Tool data"=w568, "Cutting data"=w566, "Limits"=w564, "G1 status"=w496) -> (w560:T19)
        n319 = call "Enqueue Message.vi"("Message Data"=w560, "Message"="Update Control Configuration", "Message Queue"=w572) -> ()  [unwired: 7 in, 2 out]
        n320 = case shown="True" w524 {
          tunnel: ["Plot" ("Message") "Plot and Save" ("Message")] -> w579
          tunnel: w499 -> [_ _]
          tunnel: w494 -> [_ _]
          tunnel: w497 -> [_ _]
          frame False {
          }
          frame True {
            (unwired) errorcluster {"status"=FALSE, "code"=0, "source"=""} ("error out")
          }
        }
        n321 = call "Enqueue Message.vi"("error in (no error)"=w580, "Message Data"=w578, "Message"=w579, "Message Queue"=w572) -> ("error out"=w552:errorcluster)  [unwired: 6 in, 1 out]
        n322 = call "UI Error Handler - Monitoring.vi"("error in (no error)"=w552, "Message Queue"=w600) -> ()  [unwired: 9 in, 1 out]
      }
    }
    n323 = global read "Global - All UI Loop Stop.vi" "All UI Loop Stop"() -> (w461:bool)
  }
  n324 = Unregister For Events(event registration refnum=w49, error in=w57) -> (error out=w50:errorcluster)
  n325 = Merge Errors(w50, w58) -> (w56:errorcluster)
  n326 = call "Destroy User Event - Stop.vi"("error in (no error)"=w56, "User Event - Stop"=w54) -> ("error out"=w48:errorcluster)  [unwired: 9 in]
  n327 = call <vilib>:"Simple Error Handler.vi"("error in (no error)"=w48) -> ()  [unwired: 4 in, 5 out]
